vi "FPGA DAQ.vi"() -> ()   [LabVIEW 2020]
uses:
  <vilib>/Platform/TimedLoop/XDataNode/wakeup.ctl
  <vilib>/Platform/TimedLoop/XDataNode/XDNodeRunTimeDep.lvlib
  <vilib>/Platform/TimedLoop/XDataNode/nitl_modes.ctl
  <vilib>/Platform/TimedLoop/XDataNode/timing_clust.ctl
  <vilib>/Platform/TimedLoop/XDataNode/XDataNode.xnode
  <vilib>/eio/EIONode/EIONode.xnode
  <vilib>/rvi/DataTransferAndStorage/Container/XNode/niFpgaContainer.xnode
  FPGA Typedefs/Image State.ctl
  FPGA Typedefs/scan_typr.ctl
  <vilib>/rvi/interface/RandomDataEmulation/nirviRandomDataFpgaReadWriteTemplate.vi
  FPGA Typedefs/SPI Master State.ctl
  FPGA Typedefs/first_ref_frame.ctl
  <vilib>/rvi/FXPMathLib/FxpAdd/XNode/nifxpmath_Add.xnode
  <vilib>/rvi/FXPMathLib/sim/FxpSim.dll
  <vilib>/rvi/FXPMathLib/FxpMul/XNode/nifxpmath_Multiplier.xnode
  <vilib>/rvi/FXPMathLib/FxpDiv/subVIs/nifxpmath_Div_SimConfig.ctl
  <vilib>/rvi/FXPMathLib/FxpDiv/simVIs/DllFxpDivTemp_sub.vi
  <vilib>/rvi/FXPMathLib/FxpDiv/XNode/nifxpmath_Div.xnode
  <vilib>/rvi/FXPMathLib/FxpSub/XNode/nifxpmath_Sub.xnode
  <vilib>/rvi/FIFO/Fifo_Resource/niFpgaFifoEmulationRefIn.vi
  <vilib>/rvi/FIFO/Fifo_Resource/nirvififoEmulationWrite.vi
  <vilib>/rvi/FIFO/Fifo_Resource/nirvififoEmulationGetNumberOfElementsToRead.vi
  <vilib>/rvi/eio/common/nirviEmuTemplateMethod_errors.vi
  FPGA Globals/FPGA golbals.vi
  FPGA Typedefs/Stimulus trigger delays cluster.ctl
  Typedefs/Imaging Protocols enum.ctl
  FPGA Typedefs/PXI Trigger Enable cluster.ctl
  FPGA Typedefs/General trig pulse width.ctl
  Typedefs/Trigger 1 selector enum.ctl
panel:
  in  "Trigger 1 selector":T1
  out "x_offset":fxp<+/-,16,8>
  out "MC State":T2
  out "Data Out":u32
  out "_SS":bool
  in  "live_scan (triggers module)":bool
  in  "ABORT Trig loop":bool
  in  "General trig. pulse width":T3={"Trigger 1 function"=enum."Line trigger", "Pulse width (ticks)-Line Trig."=80000, "Pulse width (ticks)-Frame/Cycle Trig."=80, "Pulse width (ticks)-Trial trig."=80, "Pulse width (ticks)-Start of Exp. trig."=80000}
  in  "Experiment start":bool
  in  "var_x":fxp<+,16,4>=1.0
  in  "var_y":fxp<+,16,4>=1.0
  in  "accn_noise":fxp<+,16,16>=3200.0
  in  "use Kalman":bool
  in  "PXI Trigger Enable":T4
  in  "Imaging Protocol":T5=enum."Live Imaging"
  in  "Stimulus Trigger Setup":T6={"Trigger period in live protocols (80MHz Cycles)"=800000000, "Pulse width in live protocols (80MHz Cycles)"=40000000, "Enable stimulus in live protocols"=FALSE, "Trigger delay in funct. protocols (80MHz Cycles)"=0, "Pulse width in funct. protocols (80MHz Cycles)"=400000, "Enable stimulus in funct. protocols"=FALSE}
  in  "New line trigger enabled":bool
  in  "Ref count reset enabled":bool
  out "x_diff_PID_out":fxp<+/-,16,8>
  out "Read Value":u32
  in  "select_ref_red":bool
  out "ydiffpidvalid":bool
  out "xpiddiffvalid":bool
  out "y_diff_PID_out":fxp<+/-,16,8>
  out "y_new_ready":bool
  out "x_new_ready":bool
  in  "scan_int":fxp<+,16,2>=0.00201416015625
  in  "Integral_scale":fxp<+/-,16,12>
  in  "diff_thresh":fxp<+/-,16,8>
  in  "proportioanl_scale":fxp<+,16,2>=1.0
  in  "live_scan":bool
  in  "start":bool
  out "x_diff":fxp<+/-,16,8>
  out "y_diff":fxp<+/-,16,8>
  out "x_centroid_ref":fxp<+,32,16>
  in  "Average":u16=1
  in  "threshold":u16
  out "y_offset_u16":u16
  out "TX ready":bool
  out "y^x offset":u32
  in  "use host offset":bool
  in  "set_reference":bool
  out "x_centroid_new":fxp<+,32,16>
  out "y_centroid_new":fxp<+,32,16>
  out "y_centroid_ref":fxp<+,32,16>
  out "y_offset":fxp<+/-,16,8>
  out "x_offset_u16":u16
  in  "x_offset_host":fxp<+/-,16,8>
  in  "y_offset_host":fxp<+/-,16,8>
  in  "scale":fxp<+,16,2>=1.0
  in  "MISO":bool
  in  "RESET":bool
  in  "CPHA":bool
  in  "CPOL":bool
  in  "HCP-1":u8
  in  "add_cycle":bool
  in  "Num_pixels_slip_cycle":u32
  in  "Repeat (Number of Cycles)":u32
  in  "Mode":T7
  in  "AOD fill":u16
  in  "Ref Scan Cycles":i32=1
  in  "Start Up Delay":i32
  in  "samps-per-pix (P)":u16=1
  in  "Number-pixels-pointing (Np)":i32
  in  "Ref y-pixels-per-line (Npyr)":i16
  in  "Ref x-pixels-per-line (Npxr)":i16
  in  "Ref samps-per-pix (Pr)":u16
  in  "y-pixels-per-line (Npy)":i16
  in  "x-pixels-per-line (Npx)":i16
  in  "samples wait after trigger":u16
  # "STATE MACHINE"
  # "TRIGGERS"
  # "HANDSHAKE"
  # "MOVEMENT CORRECTION"
  # "(Trigger 5)"
  # "Many of these indicators are used in the  PC code's MC logic (in the \"Save MC Test Data.vi\"). Their values are saved to file. Eliminate if unnecessary."
  # "(80=1us)"
  # "(80=1us)"
  # "(80000=1ms)"
  # "(80000=1ms)"
  # "Limited to 53.5 sec (if U32)"
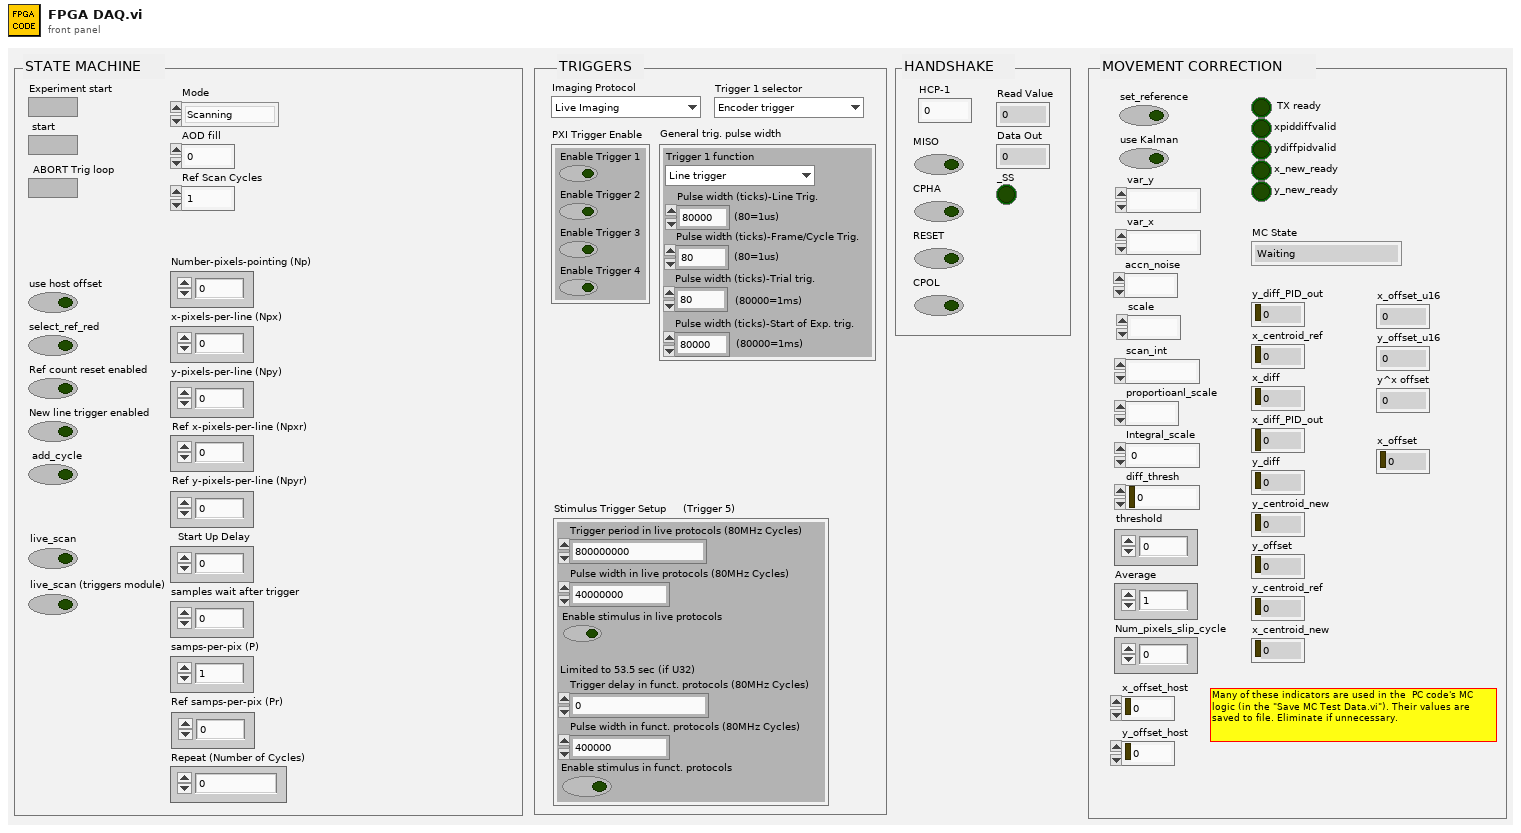
[diagram p1: front panel]
types:
  T1 = typedef "Trigger 1 selector enum.ctl" = enum16{"Encoder trigger", "Line trigger", "Control system's ref frame acknowledgement"}
  T2 = typedef "first_ref_frame.ctl" = enum16{"Waiting", "First frame", "Wrote Ref"}
  T3 = typedef "General trig pulse width.ctl" = cluster{"Trigger 1 function":T1, "Pulse width (ticks)-Line Trig.":u32, "Pulse width (ticks)-Frame/Cycle Trig.":u32, "Pulse width (ticks)-Trial trig.":u32, "Pulse width (ticks)-Start of Exp. trig.":u32}
  T4 = typedef "PXI Trigger Enable cluster.ctl" = cluster{"Enable Trigger 1":bool, "Enable Trigger 2":bool, "Enable Trigger 3":bool, "Enable Trigger 4":bool}
  T5 = typedef "Imaging Protocols enum.ctl" = enum16{"AOL Z-Stack", "Motor Z Stack", "Functional Acquisition", "Single Plane Acquisition", "Volume Acquisition", "Live Imaging", "Live Plane Imaging", "Live Volume Imaging"}
  T6 = typedef "Stimulus trigger delays cluster.ctl" = cluster{"Trigger period in live protocols (80MHz Cycles)":u32, "Pulse width in live protocols (80MHz Cycles)":u32, "Enable stimulus in live protocols":bool, "Trigger delay in funct. protocols (80MHz Cycles)":u32, "Pulse width in funct. protocols (80MHz Cycles)":u32, "Enable stimulus in funct. protocols":bool}
  T7 = typedef "scan_typr.ctl" = enum16{"Scanning", "Pointing", "Pointing & MC", "Scanning & MC"}
  T8 = typedef "Image State.ctl" = enum16{"Start Up", "Wait for Trigger", "Wait N after Trigger", "DAQ Pointing", "DAQ Scan", "Reference Scan", "Pointing AOL Fill", "Scan AOL FILL", "Reference AOL Fill"}
  T9 = typedef "XDNodeRunTimeDep.lvlib/timing_clust.ctl" = cluster{"Expected End [f-1]":u64, "Actual End [f-1]":u64, "Finished Late? [f-1]":bool, "Expected End [i-1]":u64, "Actual End [i-1]":u64, "Finished Late? [i-1]":bool, "Expected Start [i]":u64, "Actual Start [i]":u64, "Expected Start [f]":u64, "Actual Start [f]":u64, "Source Name":string, "Structure Name":string, "Period":i64, "Deadline":i64, "Offset":i64, "Start":i64, "Priority":i32, "Timeout":i32, "Mode":T10, "Wakeup Reason":T11, "Error":errorcluster, "Source Type":string, "Secondary Source Type":string, "Global End Time":u64, "Global Start Time":u64, "Frame Duration":u64, "Iteration Duration":u64, "Assigned CPU":i32, "I/O Scan Engine Mode":u32}
  T10 = typedef "XDNodeRunTimeDep.lvlib/nitl_modes.ctl" = enum32{"No Change", "Process missed periods, maintain original phase", "Discard missed periods, maintain original phase", "Process missed periods, ignore original phase", "Discard missed periods, ignore original phase"}
  T11 = typedef "XDNodeRunTimeDep.lvlib/wakeup.ctl" = enum32{"Normal", "Aborted", "Asynchronous wakeup", "Timing source error", "Timed loop error", "Timeout"}
  T12 = typedef "SPI Master State.ctl" = enum8{"RESET", "Wait for TX", "Assert MOSI", "Toggle SCLK", "Latch MISO and Toggle SCLK", "Assert MOSI and Toggle SCLK"}
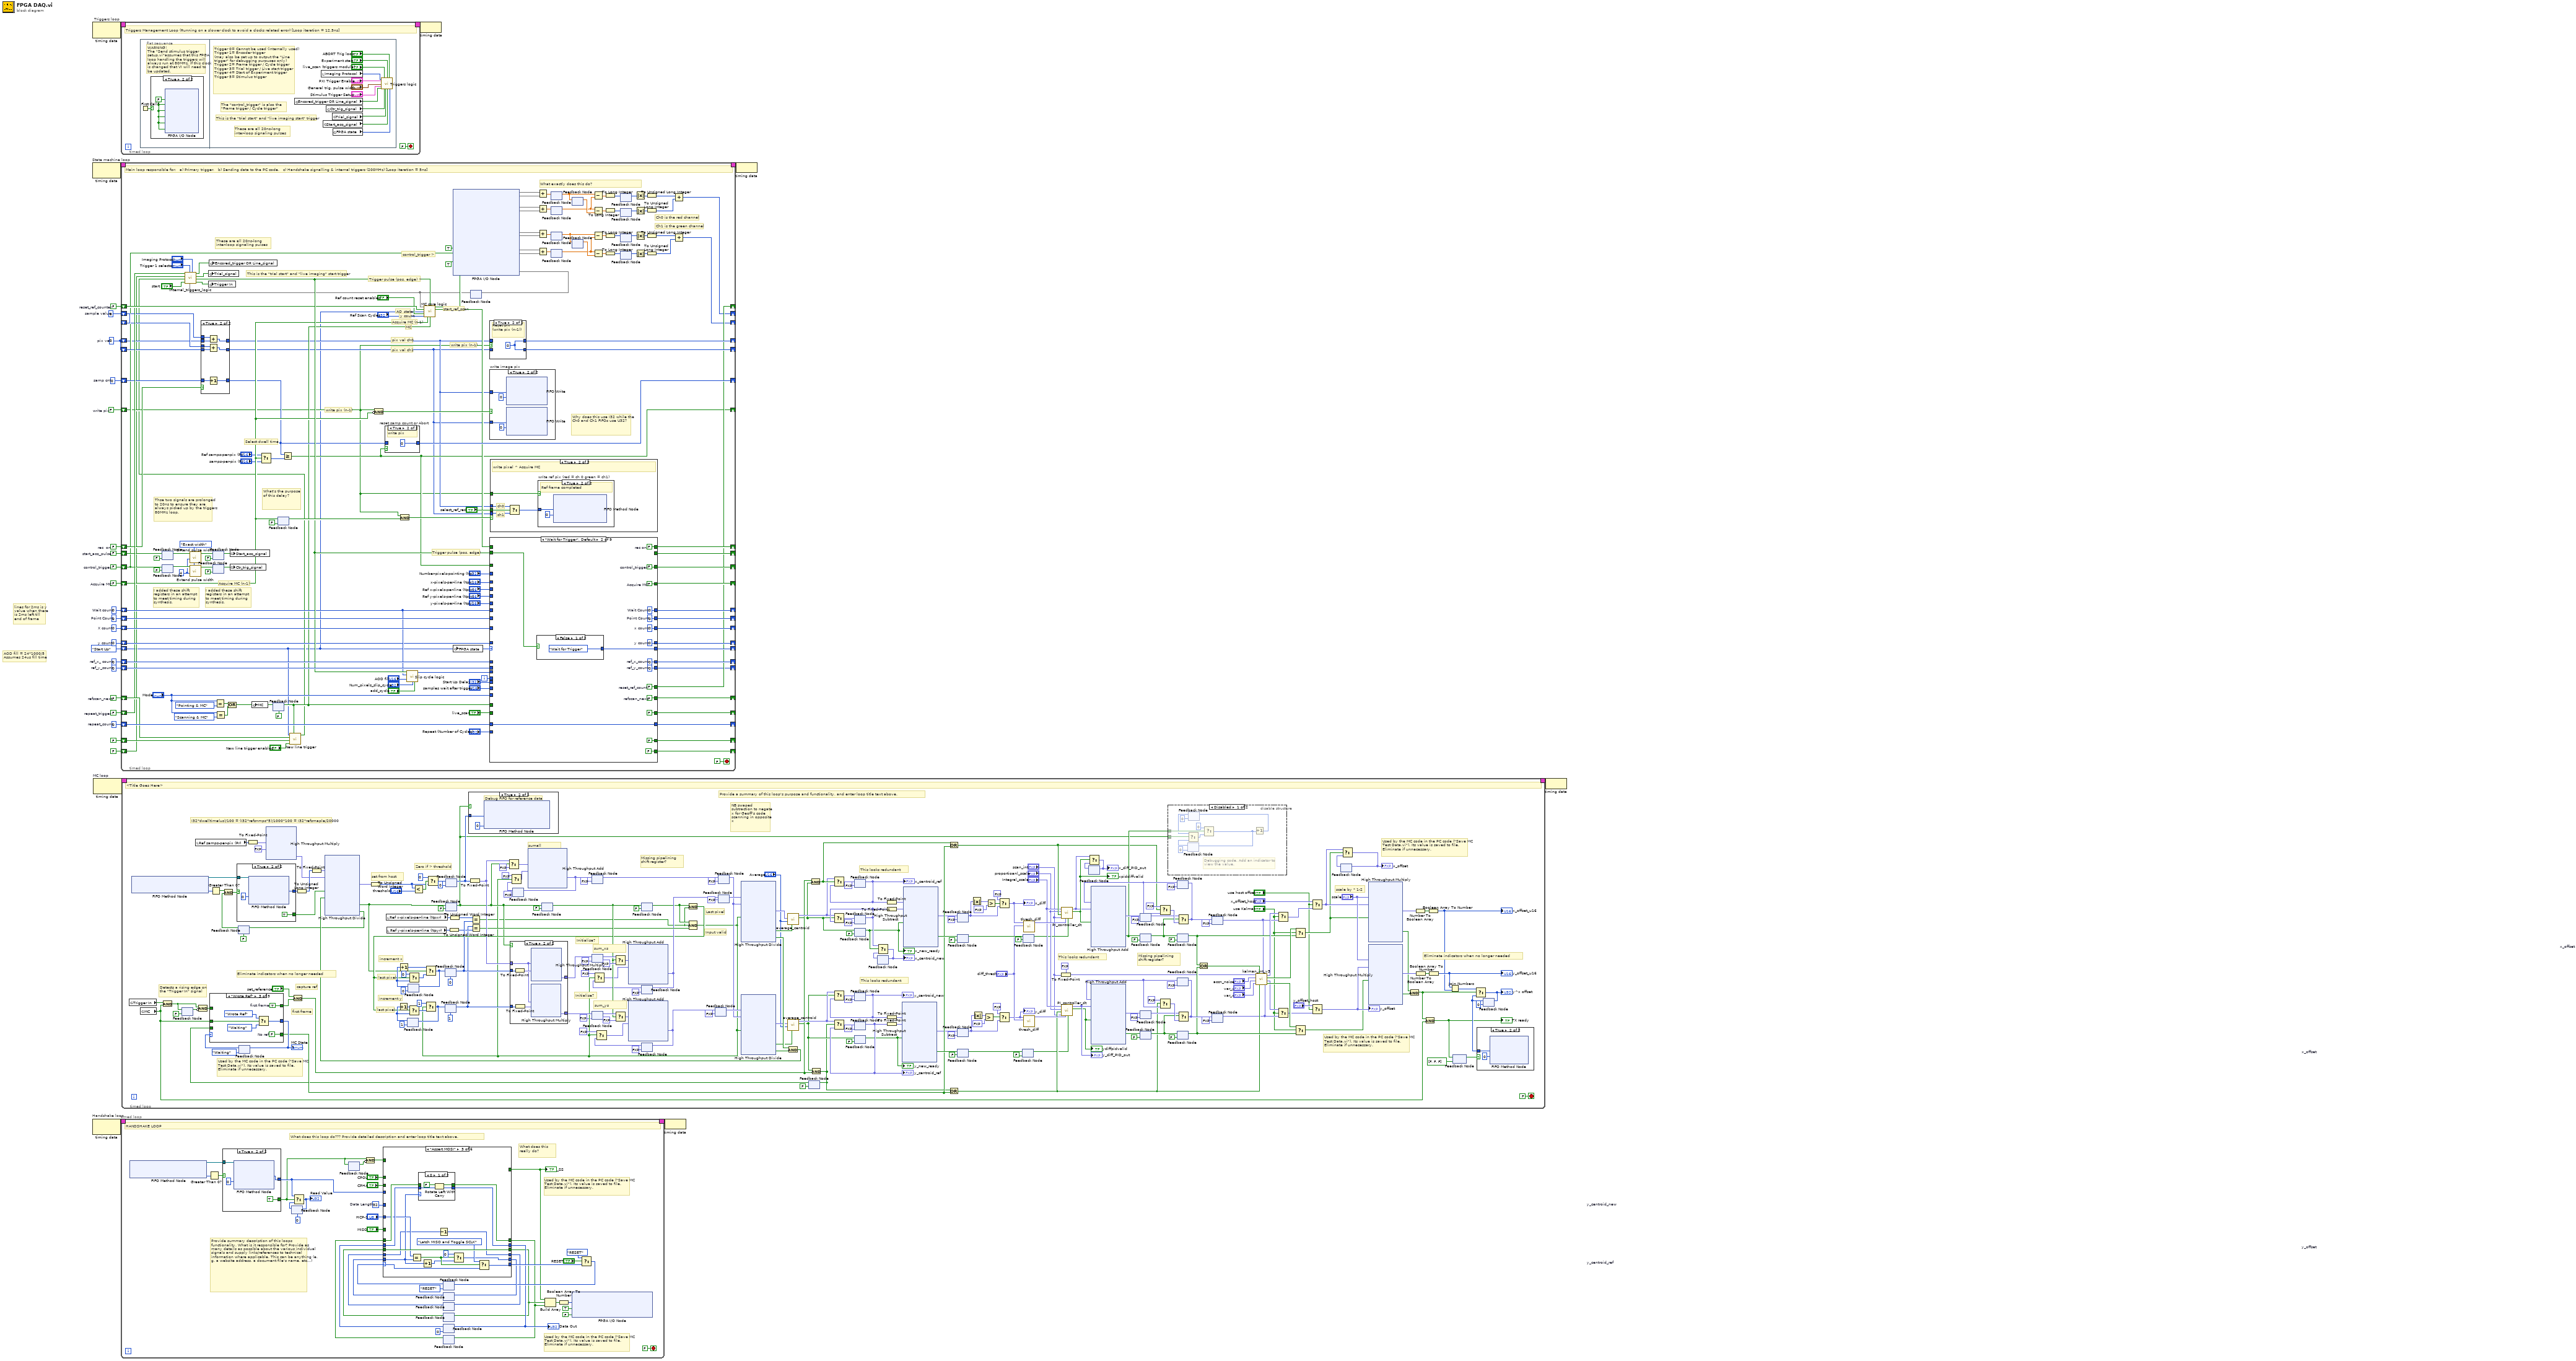
[diagram p0: block diagram]
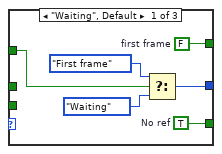
[diagram p6: hidden frame]
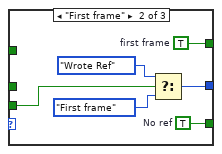
[diagram p7: hidden frame]
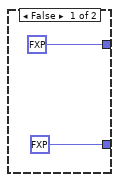
[diagram p8: hidden frame]
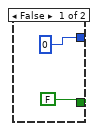
[diagram p9: hidden frame]
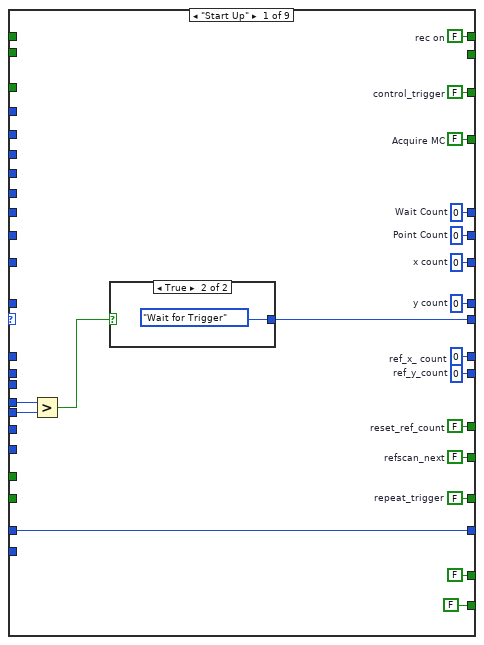
[diagram p11: hidden frame]
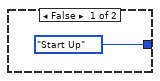
[diagram p12: hidden frame]
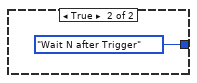
[diagram p13: hidden frame]
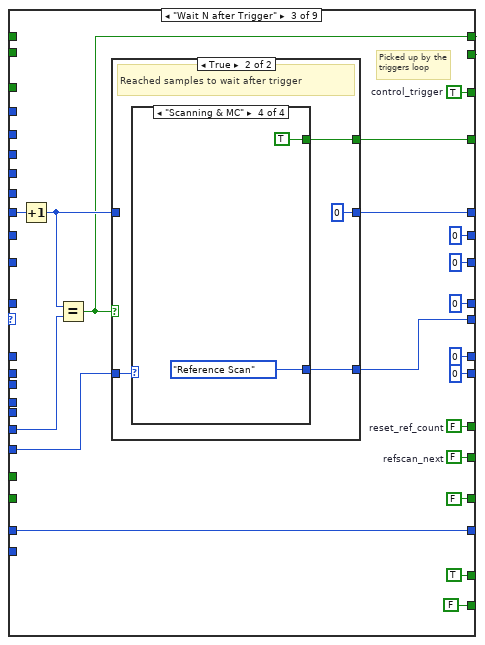
[diagram p14: hidden frame]
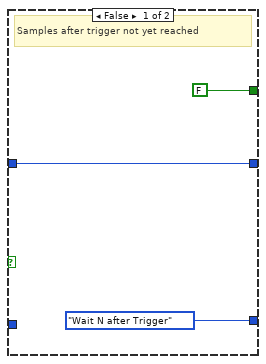
[diagram p15: hidden frame]
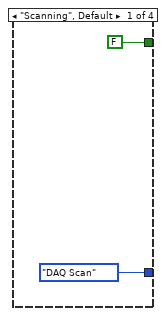
[diagram p16: hidden frame]
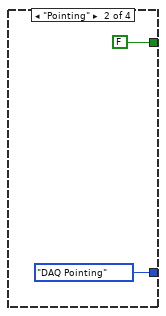
[diagram p17: hidden frame]
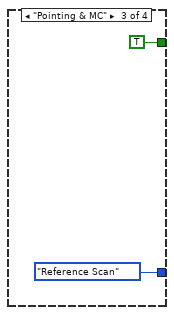
[diagram p18: hidden frame]
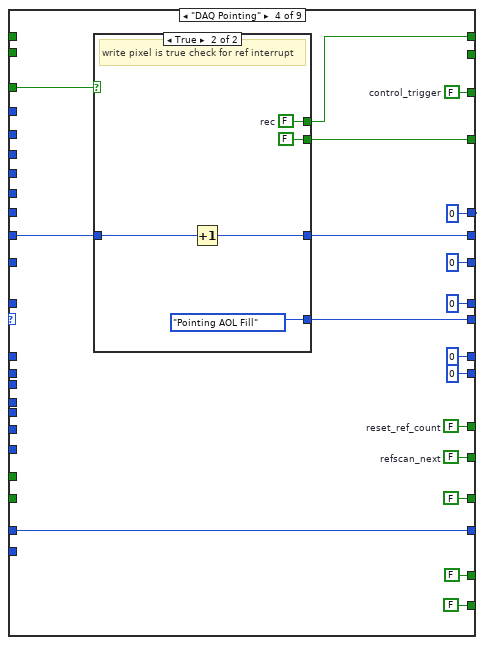
[diagram p19: hidden frame]
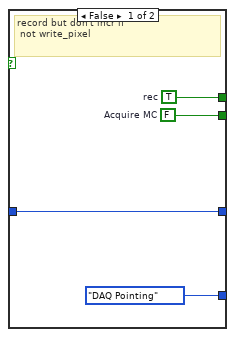
[diagram p20: hidden frame]
diagram:
  w6 = FALSE  # start_acq_pulse
  w10 = FALSE  # refscan_next
  w9 = FALSE  # reset_ref_counter
  w12 = FALSE  # repeat_trigger
  w13 = FALSE  # control_trigger
  w14 = u32 0  # repeat_count
  w16 = i16 0  # ref_y_count
  w17 = i16 0  # ref_x_ count
  w15 = u16 0  # Wait count
  w19 = FALSE  # Acquire MC
  w20 = i16 0  # y count
  w21 = i16 0  # X count
  w22 = 0  # Point Count
  w8 = FALSE  # write pix
  w7 = u32 0  # sample value
  w24 = FALSE  # rec  on
  w25 = u16 0  # samp cnt
  w23 = u32 0  # pix val
  # "lines for 2ms is y value when there is 2ms left till end of frame"
  # "AOD fill = 24*1000/5\nAssumes 24us fill time"
  n1 = node-c288() -> (w3:T9)  [unwired: 1 in]
  n2 = node-c288() -> (w27:T9)  [unwired: 1 in]
  n3 = node-c288() -> (w29:T9)  [unwired: 1 in]
  n4 = node-c288 "MC loop"() -> (w5:T9)  [unwired: 1 in]
  n5 = timed-loop "Triggers loop" {
    timing: w3 -> [_]
    timing-out: [_] -> w2
    stop <- FALSE stop-if-true
    # "Triggers Management Loop (Running on a slower clock to avoid a clocks related error) [Loop iteration = 12.5ns]"
    n6 = flat-sequence {
      frame #0 {
        # "WARNING!\nThe \"Send stimulus trigger setup.vi\"assumes that this FPGA loop handling the triggers will always run at 80MHz. If this clock is changed that VI will need to be updated."
        n7 = First Call?() -> (First Call?: T/F=w31:bool)
        n8 = case shown="True" w31 {
          frame False {
          }
          frame True {
            w32 = FALSE ("PXI_Trig0")
            n9 = xnode "FPGA I/O Node"("PXI_Trig0"=w32, "PXI_Trig1"=w32, "PXI_Trig2"=w32, "PXI_Trig3"=w32, "PXI_Trig4"=w32, "PXI_Trig5"=w32) -> ()  [unwired: 6 in, 6 out]
          }
        }
      }
      frame #1 {
        # "This is the \"trial start\" and \"live imaging start\" trigger"
        # "These are all 20ns-long inter-loop signaling pulses"
        # "The \"control_trigger\" is also the \"Frame trigger / Cycle trigger\""
        # "Trigger 0= Cannot be used (internally used)\nTrigger 1= Encoder trigger\n(may also be set up to output the \"Line trigger\" for debugging purpuses only)\nTrigger 2= Frame trigger / Cycle trigger\nTrigger 3= Trial trigger / Live start trigger\nTrigger 4= Start of Experiment trigger\nTrigger 5= Stimulus trigger"
        n10 = global read "FPGA golbals.vi" "Encored_trigger OR Line_signal"() -> (w36:bool)
        n11 = local read "Imaging Protocol"() -> (w33:T5)
        n12 = global read "FPGA golbals.vi" "Start_acq_signal"() -> (w38:bool)
        n13 = global read "FPGA golbals.vi" "Ctr_trig_signal"() -> (w37:bool)
        n14 = global read "FPGA golbals.vi" "Trial_signal"() -> (w39:bool)
        n15 = global read "FPGA golbals.vi" "FPGA state"() -> (w34:T8)
        n16 = call "Triggers logic.vi"("Imaging Protocol"=w33, "PXI Trigger Enable"="PXI Trigger Enable", "General trig. pulse width"="General trig. pulse width", "Stimulus Trigger Setup"="Stimulus Trigger Setup", "Encored_trigger OR Line_signal"=w36, "live_scan"="live_scan (triggers module)", "Ctr_trig_signal"=w37, "Trial_signal"=w39, "Experiment start"="Experiment start", "Start_acq_signal"=w38, "Abort triggers"="ABORT Trig loop", "FPGA state"=w34) -> ()  [unwired: 7 in, 1 out]
      }
    }
  }
  n17 = timed-loop "State machine loop" {
    timing: w27 -> [_]
    timing-out: [_] -> w26
    shift-right: [w191] -> _
    shift-left: w23 -> [w153]
    shift-right: [w193] -> _
    shift-left: w25 -> [w152]
    shift-right: [w100] -> _
    shift-left: w7 -> [w154]
    shift-right: [w102] -> _
    shift-left: w8 -> [w96]
    shift-right: [w130] -> _
    shift-left: w24 -> [w162]
    shift-right: [w101] -> _
    shift-left: w7 -> [w115]
    shift-right: [w192] -> _
    shift-left: w23 -> [w99]
    shift-right: [w125] -> _
    shift-left: Image_State."Start Up" ("Enum") -> [w48]
    shift-right: [w123] -> _
    shift-left: w22 -> [w188]
    shift-right: [w121] -> _
    shift-left: w21 -> [w189]
    shift-right: [w124] -> _
    shift-left: w20 -> [w164]
    shift-right: [w128] -> _
    shift-left: w19 -> [w137]
    shift-right: [w126] -> _
    shift-left: w17 -> [w186]
    shift-right: [w111] -> _
    shift-left: w16 -> [w187]
    shift-right: [w122] -> _
    shift-left: w15 -> [w166]
    shift-right: [w117] -> _
    shift-left: w14 -> [w181]
    shift-right: [w129] -> _
    shift-left: w13 -> [w108]
    shift-right: [w118] -> _
    shift-left: w12 -> [w163]
    shift-right: [w116] -> _
    shift-left: FALSE -> [w177]
    shift-right: [w120] -> _
    shift-left: w9 -> [w165]
    shift-right: [w119] -> _
    shift-left: w10 -> [w178]
    shift-right: [w127] -> _
    shift-left: w6 -> [w160]
    shift-right: [w55] -> _
    shift-left: FALSE -> [w53]
    i -> [w190]
    stop <- FALSE stop-if-true
    w161 = enum16{"Minimum width", "Exact width"}."Exact width" ("Function")
    w151 = u32 4 ("Pulse width (ticks)(80000=1ms @80MHz)")
    # "These are all 20ns-long inter-loop signaling pulses"
    # "This is the \"trial start\" and \"live imaging\" start trigger"
    # "What exactly does this do?"
    # "Ch1 is the green channel"
    # "Ch0 is the red channel"
    # "write pix (n-1)"
    # "pix val ch1"
    # "pix val ch0"
    # "control_trigger >"
    # "What's the purpose of this delay?"
    # "write pix (n-1)"
    # "Why does this use I32 while the Ch0 and Ch1 FIFOs use U32?"
    # "Select dwell time"
    # "Trigger pulse (pos. edge)"
    # "I added these shift registers in an attempt to meet timing during synthesis."
    # "I added these shift registers in an attempt to meet timing during synthesis."
    # "Thse two signals are prolonged to 20ns to ensure they are always picked up by the triggers 80MHz loop."
    # "MC"
    # "AQ_state"
    # "Trigger pulse (pos. edge) >"
    # "Acquire MC (n-1)"
    # "start_ref_scan"
    # "Acquire MC (n-1)"
    # "y count"
    # "Main loop responsible for:   a) Primary trigger,   b) Sending data to the PC code,   c) Handshake signalling & internal triggers (200MHz) [Loop iteration = 5ns]"
    n18 = feedback #1(FALSE ("Acquire MC")) -> (w159:bool)
    n19 = feedback-in #1(w160) -> ()
    n20 = feedback #2(FALSE ("Acquire MC")) -> (w158:bool)
    n21 = feedback-in #2(w108) -> ()
    n22 = call "Extend pulse width.vi"("Function"=w161, "Pulse width (ticks)(80000=1ms @80MHz)"=w151, "Input signal"=w159) -> ("Output signal"=w157:bool)  [unwired: 8 in]
    n23 = call "Extend pulse width.vi"("Function"=w161, "Pulse width (ticks)(80000=1ms @80MHz)"=w151, "Input signal"=w158) -> ("Output signal"=w156:bool)  [unwired: 8 in]
    n24 = case shown="True" w162 {
      tunnel: w153 -> [w196 w204]
      tunnel: [w196 w203] -> w97
      tunnel: w152 -> [w195 w202]
      tunnel: [w195 w201] -> w113
      tunnel: w154 -> [_ w200]
      tunnel: w99 -> [w194 w199]
      tunnel: w115 -> [_ w198]
      tunnel: [w194 w197] -> w98
      frame False {
      }
      frame True {
        n25 = Add(x=w198, y=w199) -> (x+y=w197:u32)
        n26 = Add(x=w200, y=w204) -> (x+y=w203:u32)
        n27 = Increment(x=w202) -> (x+1=w201:u16)
      }
    }
    n28 = feedback #3(FALSE ("Acquire MC")) -> (w105:bool)
    n29 = feedback-in #3(w157) -> ()
    n30 = feedback #4(FALSE ("Acquire MC")) -> (w104:bool)
    n31 = feedback-in #4(w156) -> ()
    n32 = Equal?(x="Mode", y=scan_typr."Pointing & MC" ("Mode 2")) -> (x = y?=w183:bool)
    n33 = Equal?(x="Mode", y=scan_typr."Scanning & MC" ("Mode 2")) -> (x = y?=w182:bool)
    n34 = Or(x=w183, y=w182) -> (x .or. y?=w103:bool)
    n35 = global write "FPGA golbals.vi" "Start_acq_signal"(w105) -> ()
    n36 = global write "FPGA golbals.vi" "Ctr_trig_signal"(w104) -> ()
    n37 = global write "FPGA golbals.vi" "MC"(w103) -> ()
    n38 = Select(t="Ref samps-per-pix (Pr)", s=w137, f="samps-per-pix (P)") -> (s? t:f=w114:u16)
    n39 = feedback-in #5(w103) -> ()
    n40 = feedback #5(FALSE ("Acquire MC")) -> (w112:bool)
    n41 = feedback #6(FALSE ("Acquire MC")) -> (w174:bool)
    n42 = feedback-in #6(w137) -> ()
    n43 = Greater Or Equal?(x=w113, y=w114) -> (x >= y?=w102:bool)
    n44 = call "New line trigger.vi"("MC"=w112, "New line trigger enabled"="New line trigger enabled", "aod_fill_active in"=w177, "refscan_next"=w178, "AQ STATE"=w48) -> ("aod_fill_active"=w51:bool)  [unwired: 6 in]
    n45 = Compound Arithmetic op=AND(w96, invert w137) -> (w179:bool)
    n46 = case "reset samp count or Abort" shown="True" w102 {
      tunnel: [w609 u16 0] -> w193
      tunnel: w113 -> [w609 _]
      frame False {
      }
      frame True {
        # "write pix"
      }
    }
    n47 = And(x=w96, y=w174) -> (x .and. y?=w173:bool)
    n48 = global write "FPGA golbals.vi" "FPGA state"(w48) -> ()
    n49 = feedback #7() -> (w49)  [unwired: 1 in]
    n50 = call "Internal_triggers_logic.vi"("Imaging Protocol"="Imaging Protocol", "aol_ref_scan_next"=w49, "Trigger 1 selector"="Trigger 1 selector", "Start"="start", "Line_signal"=w51, "End of trial"=w53, "Repeat trigger"=w163) -> ("Trigger In"=w106:bool, "Trigger pulse (pos. edge)"=w169:bool, "Trial start trigger signal"=w107:bool, "Encoder trigger signal"=w52:bool)  [unwired: 1 in]
    n51 = global write "FPGA golbals.vi" "Trial_signal"(w107) -> ()
    n52 = global write "FPGA golbals.vi" "Trigger In"(w106) -> ()
    n53 = global write "FPGA golbals.vi" "Encored_trigger OR Line_signal"(w52) -> ()
    n54 = call "Slip cycle logic.vi"("Trigger pulse (pos. edge)"=w169, "Wait Count"=w166, "AOD fill in"="AOD fill", "Num_pixels_slip_cycle"="Num_pixels_slip_cycle", "add_cycle"="add_cycle") -> ("AOD fill out"=w171:u16)  [unwired: 10 in]
    n55 = call "MC core logic.vi"("AOL_ref_scan_next"=w49, "Trigger pulse (pos. edge)"=w169, "Reset_ref_counter"=w165, "State"=w48, "Ref count reset enabled"="Ref count reset enabled", "Ref Scan Cycles"="Ref Scan Cycles", "Acquire MC"=w137, "MC"=w112) -> ("start_aol_ref_scan"=w109:bool, "start_ref_scan"=w131:bool)  [unwired: 6 in]
    n56 = xnode ("FPGA I/O Node")("IO Module\\Trigger WE"=TRUE ("IO Module\\Trigger WE"), "IO Module\\Trigger Output"=w108, "IO Module\\PFI 0 Wr Data"=w109, "IO Module\\PFI 0 WE"=TRUE ("IO Module\\PFI 0 WE")) -> ("IO Module\\AI 0 Data N"=w93, "IO Module\\AI 0 Data N-1"=w92, "IO Module\\AI 0 Data N-2"=w91, "IO Module\\AI 0 Data N-3"=w90, "IO Module\\AI 1 Data N"=w89, "IO Module\\AI 1 Data N-1"=w88, "IO Module\\AI 1 Data N-2"=w87, "IO Module\\AI 1 Data N-3"=w86, "IO Module\\PFI 1 Rd Data"=w110)  [unwired: 13 in, 13 out]
    n57 = feedback-in #7(w110) -> ()
    n58 = case shown="True" w96 {
      tunnel: [w612 w613] -> w191
      tunnel: w97 -> [w612 _]
      tunnel: w98 -> [w611 _]
      tunnel: [w611 w613] -> w192
      frame False {
      }
      frame True {
        w613 = u32 0
        # "Reset pix\n(write pix (n-1))"
      }
    }
    n59 = case "write image pix" shown="True" w179 {
      tunnel: w98 -> [_ w608]
      tunnel: w97 -> [_ w606]
      frame False {
      }
      frame True {
        n60 = xnode ("FIFO Write")("Element"=w608, "Timeout"=0) -> ()  [unwired: 1 in, 2 out]
        n61 = xnode ("FIFO Write")("Element"=w606, "Timeout"=0) -> ()  [unwired: 1 in, 2 out]
      }
    }
    n62 = case shown="\"Wait for Trigger\", Default" w48 {
      tunnel: w190 -> [w223 _ _ _ _ _ _ _ _]
      tunnel: "Start Up Delay" -> [w222 _ _ _ _ _ _ _ _]
      tunnel: [w220 w237 w262 w288 w323 w376 w439 w508 w569] -> w125
      tunnel: [w219 w241 w246 w289 w318 w378 w438 w507 w565] -> w130
      tunnel: [w218 w240 0 ("x count") w291 0 ("x count") w361 w432 0 ("x count") w567] -> w123
      tunnel: w188 -> [_ _ _ w292 _ w362 w423 _ w567]
      tunnel: [w217 w239 i16 0 i16 0 ("x count") w321 w359 i16 0 ("x count") w492 w574] -> w121
      tunnel: w189 -> [_ _ _ _ w319 w360 _ w493 w574]
      tunnel: [w216 w238 i16 0 i16 0 ("y count") w322 w357 i16 0 ("y count") w501 w570] -> w124
      tunnel: w164 -> [_ _ _ _ w320 w358 _ w490 w570]
      tunnel: [w215 w242 w247 w290 w317 w356 w437 w506 w564] -> w128
      tunnel: "samples wait after trigger" -> [_ _ w264 _ _ _ _ _ _]
      tunnel: "Mode" -> [_ _ w259 _ _ _ _ _ w563]
      tunnel: w169 -> [_ w236 _ _ _ _ _ _ _]
      tunnel: "Number-pixels-pointing (Np)" -> [_ _ _ _ _ _ w424 _ _]
      tunnel: w112 -> [_ _ _ _ _ _ w434 w503 _]
      tunnel: [w214 w235 w258 u16 0 ("Wait Count") u16 0 ("Wait count") u16 0 ("Wait count") w442 w511 w573] -> w122
      tunnel: w171 -> [_ _ _ _ _ _ w443 w510 w572]
      tunnel: w131 -> [_ _ _ _ _ _ w433 w502 _]
      tunnel: "x-pixels-per-line (Npx)" -> [_ _ _ _ w310 _ _ _ _]
      tunnel: "y-pixels-per-line (Npy)" -> [_ _ _ _ _ _ _ w491 _]
      tunnel: "Ref x-pixels-per-line (Npxr)" -> [_ _ _ _ _ w364 _ _ _]
      tunnel: "Ref y-pixels-per-line (Npyr)" -> [_ _ _ _ _ _ _ _ w557]
      tunnel: [w213 w234 i16 0 ("Wait count") i16 0 ("Wait count") i16 0 ("Wait count") w374 i16 0 ("ref_x_count") i16 0 ("ref_x_count") w568] -> w126
      tunnel: [w212 w233 i16 0 ("ref_y_count") i16 0 ("ref_y_count") i16 0 ("ref_y_count") w373 i16 0 ("ref_y_count") i16 0 ("ref_y_count") w556] -> w111
      tunnel: w187 -> [_ _ _ _ _ w372 _ _ w556]
      tunnel: w186 -> [_ _ _ _ _ w371 _ _ w568]
      tunnel: w166 -> [_ _ w254 _ _ _ w417 w488 w554]
      tunnel: "Repeat (Number of Cycles)" -> [_ _ _ _ _ _ w421 w486 _]
      tunnel: w181 -> [w211 w232 w253 w287 w316 w370 w418 w484 w566]
      tunnel: [w211 w232 w253 w287 w316 w370 w431 w500 w566] -> w117
      tunnel: [w210 w231 w252 w286 w315 w369 w430 w499 w562] -> w129
      tunnel: [w209 FALSE FALSE FALSE FALSE FALSE w429 w498 FALSE] -> w118
      tunnel: "live_scan" -> [_ _ _ _ _ _ w428 w497 _]
      tunnel: [FALSE FALSE TRUE FALSE FALSE FALSE TRUE TRUE TRUE] -> w116
      tunnel: [w207 w228 w249 w283 w312 w366 w426 w495 w559] -> w120
      tunnel: [w206 w227 w248 w282 w311 w365 w425 w494 w558] -> w119
      tunnel: [_ _ w246 _ _ _ _ _ _] -> w127
      tunnel: w102 -> [_ _ _ w281 w308 w355 _ _ _]
      tunnel: [FALSE FALSE FALSE FALSE FALSE FALSE w415 w482 FALSE] -> w55
      frame "Start Up" {
        w206 = FALSE  # refscan_next
        w207 = FALSE  # reset_ref_count
        w209 = FALSE  # repeat_trigger
        w210 = FALSE  # control_trigger
        w212 = i16 0  # ref_y_count
        w213 = i16 0  # ref_x_ count
        w214 = u16 0  # Wait Count
        w215 = FALSE  # Acquire MC
        w216 = i16 0  # y count
        w217 = i16 0  # x count
        w219 = FALSE  # rec on
        w218 = 0  # Point Count
        n63 = Greater?(x=w223, y=w222) -> (0:w221:bool)
        n64 = case shown="True" w221 {
          tunnel: [Image_State."Start Up" Image_State."Wait for Trigger"] -> w220
          frame False {
          }
          frame True {
          }
        }
      }
      frame "Wait for Trigger", Default {
        w227 = FALSE  # refscan_next
        w228 = FALSE  # reset_ref_count
        w231 = FALSE  # control_trigger
        w233 = i16 0  # ref_y_count
        w234 = i16 0  # ref_x_count
        w235 = u16 0  # Wait Count
        w242 = FALSE  # Acquire MC
        w238 = i16 0  # y count
        w239 = i16 0  # x count
        w241 = FALSE  # rec on
        w240 = 0  # Point Count
        n65 = case shown="False" w236 {
          tunnel: [Image_State."Wait for Trigger" Image_State."Wait N after Trigger"] -> w237
          frame False {
          }
          frame True {
          }
        }
      }
      frame "Wait N after Trigger" {
        w248 = FALSE  # refscan_next
        w249 = FALSE  # reset_ref_count
        w252 = TRUE  # control_trigger
        # "Picked up by the triggers loop"
        # "time includes AOD fill time"
        n66 = Increment(x=w254) -> (x+1=w263:u16)
        n67 = Equal?(x=w263, y=w264) -> (x = y?=w246:bool)
        n68 = case shown="True" w246 {
          tunnel: w263 -> [w267 _]
          tunnel: [w267 u16 0] -> w258
          tunnel: [Image_State."Wait N after Trigger" w269] -> w262
          tunnel: [FALSE w270] -> w247
          tunnel: w259 -> [_ w268]
          frame False {
            # "Samples after trigger not yet reached"
          }
          frame True {
            # "Reached samples to wait after trigger"
            n69 = case shown="\"Scanning & MC\"" w268 {
              tunnel: [FALSE FALSE TRUE TRUE] -> w270
              tunnel: [Image_State."DAQ Scan" Image_State."DAQ Pointing" Image_State."Reference Scan" Image_State."Reference Scan"] -> w269
              frame "Scanning", Default {
              }
              frame "Pointing" {
              }
              frame "Pointing & MC" {
              }
              frame "Scanning & MC" {
              }
            }
          }
        }
      }
      frame "DAQ Pointing" {
        w282 = FALSE  # refscan_next
        w283 = FALSE  # reset_ref_count
        w286 = FALSE  # control_trigger
        n70 = case shown="True" w281 {
          tunnel: [Image_State."DAQ Pointing" ("Enum") Image_State."Pointing AOL Fill" ("Enum")] -> w288
          tunnel: [w300 w306] -> w289
          tunnel: [w298 w305] -> w291
          tunnel: [w299 FALSE] -> w290
          tunnel: w292 -> [w298 w304]
          frame False {
            w299 = FALSE  # Acquire MC
            w300 = TRUE  # rec
            # "record but don't incr if \n not write_pixel"
          }
          frame True {
            w306 = FALSE  # rec
            # "write pixel is true check for ref interrupt"
            n71 = Increment(x=w304) -> (x+1=w305:i32)
          }
        }
      }
      frame "DAQ Scan" {
        w311 = FALSE  # refscan_next
        w312 = FALSE  # reset_ref_count
        w315 = FALSE  # control_trigger
        n72 = Decrement(x=w310) -> (x-1=w309:i16)
        n73 = Equal?(x=w309, y=w319) -> (x = y?=w324:bool)
        n74 = case shown="True" w308 {
          tunnel: [w333 w336] -> w318
          tunnel: [FALSE w335] -> w317
          tunnel: w319 -> [w331 w341]
          tunnel: [w331 w340] -> w321
          tunnel: w320 -> [w330 w339]
          tunnel: [w330 w338] -> w322
          tunnel: [Image_State."DAQ Scan" ("Enum") w337] -> w323
          tunnel: w324 -> [_ w334]
          frame False {
            w333 = TRUE  # rec
            # "accumulate samples for pixel"
          }
          frame True {
            # "write pixel check for  end of line"
            n75 = case shown="True" w334 {
              tunnel: w341 -> [w347 _]
              tunnel: [w346 w353] -> w340
              tunnel: w339 -> [w345 w352]
              tunnel: [w345 w351] -> w338
              tunnel: [Image_State."DAQ Scan" ("Enum") Image_State."Scan AOL FILL" ("Enum")] -> w337
              tunnel: [w343 w350] -> w336
              tunnel: [w342 w349] -> w335
              frame False {
                w342 = FALSE  # Acq MC
                w343 = TRUE  # rec
                # "not end of line"
                n76 = Increment(x=w347) -> (x+1=w346:i16)
              }
              frame True {
                w349 = FALSE  # Acquire MC
                w350 = FALSE  # rec
                w353 = i16 0  # x count
                # "End of line"
                n77 = Increment(x=w352) -> (x+1=w351:i16)
              }
            }
          }
        }
      }
      frame "Reference Scan" {
        w356 = TRUE  # Acq MC
        w365 = FALSE  # refscan_next
        w366 = FALSE  # reset_ref_count
        w369 = FALSE  # control_trigger
        n78 = Decrement(x=w364) -> (x-1=w363:i16)
        n79 = Equal?(x=w363, y=w371) -> (x = y?=w375:bool)
        n80 = case shown="True" w355 {
          tunnel: [w385 w396] -> w378
          tunnel: [Image_State."Reference Scan" ("Enum") w397] -> w376
          tunnel: w375 -> [_ w398]
          tunnel: w371 -> [w383 w395]
          tunnel: [w383 w394] -> w374
          tunnel: w372 -> [w382 w393]
          tunnel: [w382 w392] -> w373
          tunnel: w362 -> [w381 w391]
          tunnel: [w381 w390] -> w361
          tunnel: w360 -> [w380 w389]
          tunnel: [w380 w388] -> w359
          tunnel: w358 -> [w379 w387]
          tunnel: [w379 w386] -> w357
          frame False {
            w385 = TRUE  # rec
            # "accumulate samples for pixel"
          }
          frame True {
            # "write pixel check for  end of line"
            n81 = case shown="False" w398 {
              tunnel: [w406 i16 0] -> w394
              tunnel: [Image_State."Reference Scan" ("Enum") Image_State."Reference AOL Fill" ("Enum")] -> w397
              tunnel: [w405 w410] -> w396
              tunnel: w395 -> [w404 _]
              tunnel: w393 -> [w403 w413]
              tunnel: [w403 w412] -> w392
              tunnel: [w401 w409] -> w390
              tunnel: w391 -> [w401 w409]
              tunnel: [w400 w408] -> w388
              tunnel: w389 -> [w400 w408]
              tunnel: [w399 w407] -> w386
              tunnel: w387 -> [w399 w407]
              frame False {
                w405 = TRUE  # rec
                # "not end of line"
                n82 = Increment(x=w404) -> (x+1=w406:i16)
              }
              frame True {
                w410 = FALSE  # rec
                # "end of line - AOL Fill"
                n83 = Increment(x=w413) -> (x+1=w412:i16)
              }
            }
          }
        }
      }
      frame "Pointing AOL Fill" {
        w430 = FALSE  # control_trigger
        n84 = And(x=w433, y=w434) -> (x .and. y?=w425:bool)
        n85 = Equal?(x=w424, y=w423) -> (x = y?=w422:bool)
        n86 = Equal?(x=w417, y=w443) -> (x = y?=w438:bool)
        n87 = Increment(x=w418) -> (x+1=w419:u32)
        n88 = Greater Or Equal?(x=w418, y=w421) -> (x >= y?=w420:bool)
        n89 = Increment(x=w417) -> (x+1=w416:u16)
        n90 = case shown="True" w438 {
          tunnel: [w464 w475] -> w442
          tunnel: [w462 w472] -> w439
          tunnel: [FALSE ("Acquire MC") w474] -> w437
          tunnel: w425 -> [_ w473]
          tunnel: w416 -> [w445 _]
          tunnel: w423 -> [w449 w471]
          tunnel: [w460 w471] -> w432
          tunnel: w421 -> [_ _]
          tunnel: w418 -> [w457 w470]
          tunnel: [w458 w470] -> w431
          tunnel: [w450 FALSE] -> w429
          tunnel: w428 -> [w455 _]
          tunnel: [w452 w468] -> w426
          tunnel: w422 -> [w448 _]
          tunnel: w420 -> [w447 _]
          tunnel: w419 -> [w446 _]
          tunnel: [w444 FALSE] -> w415
          frame False {
            w452 = FALSE  # reset_ref_count
            # "counting AOD fill time and check for last"
            n91 = Select(t=w446, s=w448, f=w457) -> (s? t:f=w456:u32)
            n92 = Compound Arithmetic op=AND(w448, w455) -> (w454:bool)
            n93 = Compound Arithmetic op=AND(w448, invert w447) -> (w453:bool)
            n94 = Compound Arithmetic op=AND(w448, w447) -> (w444:bool)
            n95 = Or(x=w454, y=w453) -> (x .or. y?=w450:bool)
            n96 = Select(t=u32 0, s=w444, f=w456) -> (s? t:f=w458:u32)
            n97 = Select(t=Image_State."Wait for Trigger" ("Enum"), s=w448, f=Image_State."Pointing AOL Fill" ("Enum")) -> (s? t:f=w462:T8)
            n98 = Select(t=u16 0, s=w448, f=w445) -> (s? t:f=w464:u16)
            n99 = Select(t=0, s=w448, f=w449) -> (s? t:f=w460:i32)
          }
          frame True {
            w475 = u16 0  # Wait count
            # "AOD fill time reached check to see if ref scan interrupt"
            n100 = case shown="True" w473 {
              tunnel: [Image_State."DAQ Pointing" ("Enum") Image_State."Reference Scan" ("Enum")] -> w472
              tunnel: [FALSE ("Acquire MC") TRUE ("Acquire MC")] -> w474
              tunnel: [w476 w479] -> w468
              frame False {
                w476 = FALSE  # reset_ref_count
              }
              frame True {
                w479 = TRUE  # reset_ref_count
                # "scan interrupt\nset AcquireMC"
              }
            }
          }
        }
      }
      frame "Scan AOL FILL" {
        w499 = FALSE  # control_trigger
        n101 = And(x=w502, y=w503) -> (x .and. y?=w494:bool)
        n102 = Increment(x=w488) -> (x+1=w487:u16)
        n103 = Equal?(x=w491, y=w490) -> (x = y?=w489:bool)
        n104 = Equal?(x=w488, y=w510) -> (x = y?=w507:bool)
        n105 = Increment(x=w484) -> (x+1=w483:u32)
        n106 = Greater Or Equal?(x=w484, y=w486) -> (x >= y?=w485:bool)
        n107 = case shown="True" w507 {
          tunnel: [w531 w545] -> w511
          tunnel: [w534 w544] -> w508
          tunnel: w494 -> [_ w543]
          tunnel: [w535 w542] -> w506
          tunnel: w487 -> [w516 _]
          tunnel: w490 -> [w518 w541]
          tunnel: [w530 w541] -> w501
          tunnel: w484 -> [w520 w540]
          tunnel: w486 -> [_ _]
          tunnel: [w526 w540] -> w500
          tunnel: [w519 w539] -> w498
          tunnel: w497 -> [w524 _]
          tunnel: [w521 w538] -> w495
          tunnel: w493 -> [w517 w537]
          tunnel: [w517 w537] -> w492
          tunnel: w489 -> [w515 _]
          tunnel: w485 -> [w514 _]
          tunnel: w483 -> [w513 _]
          tunnel: [w512 FALSE] -> w482
          frame False {
            w521 = FALSE  # reset_ref_count
            w535 = FALSE  # Acquire MC
            # "counting AOD fill time and check finished last line"
            n108 = And(x=w515, y=w514) -> (x .and. y?=w512:bool)
            n109 = And(x=w515, y=w524) -> (x .and. y?=w523:bool)
            n110 = Compound Arithmetic op=AND(w515, invert w514) -> (w522:bool)
            n111 = Or(x=w523, y=w522) -> (x .or. y?=w519:bool)
            n112 = Select(t=Image_State."Wait for Trigger" ("Enum"), s=w515, f=Image_State."Scan AOL FILL" ("Enum")) -> (s? t:f=w534:T8)
            n113 = Select(t=w513, s=w515, f=w520) -> (s? t:f=w527:u32)
            n114 = Select(t=u16 0, s=w515, f=w516) -> (s? t:f=w531:u16)
            n115 = Select(t=i16 0, s=w515, f=w518) -> (s? t:f=w530:i16)
            n116 = Select(t=u32 0, s=w512, f=w527) -> (s? t:f=w526:u32)
          }
          frame True {
            w539 = FALSE  # repeat_trigger
            w545 = u16 0  # Wait count
            # "AOD fill time reached check to see if ref scan interrupt"
            n117 = case shown="True" w543 {
              tunnel: [Image_State."DAQ Scan" ("Enum") Image_State."Reference Scan" ("Enum")] -> w544
              tunnel: [w548 w550] -> w542
              tunnel: [w546 w549] -> w538
              frame False {
                w546 = FALSE  # reset_ref_count
                w548 = FALSE  # Acquire MC
                # "resume scan"
              }
              frame True {
                w549 = TRUE  # reset_ref_count
                w550 = TRUE  # Acquire MC
                # "scan interrupt\nset AcquireMC"
              }
            }
          }
        }
      }
      frame "Reference AOL Fill" {
        w558 = FALSE  # refscan_next
        w559 = FALSE  # reset_ref_count
        w562 = FALSE  # control_trigger
        n118 = Equal?(x=w554, y=w572) -> (x = y?=w571:bool)
        n119 = Equal?(x=w557, y=w556) -> (x = y?=w555:bool)
        n120 = Increment(x=w554) -> (x+1=w553:u16)
        n121 = case shown="True" w571 {
          tunnel: [w575 w584] -> w573
          tunnel: [Image_State."Reference AOL Fill" ("Enum") w583] -> w569
          tunnel: w553 -> [w575 _]
          tunnel: [w577 w582] -> w565
          tunnel: [TRUE w581] -> w564
          tunnel: w563 -> [_ w580]
          tunnel: w555 -> [_ w579]
          frame False {
            w577 = FALSE  # rec
            # "counting AOD fill time"
          }
          frame True {
            w582 = TRUE  # rec
            w584 = u16 0  # Wait count
            # "AOD fill time reached"
            n122 = case shown="True" w579 {
              tunnel: [Image_State."Reference Scan" ("Enum") w587] -> w583
              tunnel: [TRUE ("Acquire MC") w588] -> w581
              tunnel: w580 -> [_ w589]
              frame False {
              }
              frame True {
                n123 = case shown="\"Pointing & MC\"" w589 {
                  tunnel: [Image_State."DAQ Scan" ("Enum") Image_State."DAQ Pointing" ("Enum") Image_State."DAQ Pointing" ("Enum") Image_State."DAQ Scan" ("Enum")] -> w587
                  tunnel: [FALSE FALSE FALSE FALSE] -> w588
                  frame "Scanning", Default {
                  }
                  frame "Pointing" {
                  }
                  frame "Pointing & MC" {
                  }
                  frame "Scanning & MC" {
                  }
                }
              }
            }
          }
        }
      }
    }
    n124 = case shown="True" w173 {
      tunnel: w98 -> [_ w602]
      tunnel: w97 -> [_ w601]
      tunnel: "select_ref_red" -> [_ w600]
      tunnel: w96 -> [_ w598]
      frame False {
      }
      frame True {
        # "ch1"
        # "ch0"
        # "write pixel ^ Acquire MC"
        n125 = Select(t=w602, s=w600, f=w601) -> (s? t:f=w599:u32)
        n126 = case "write ref pix (red = ch 0 green = ch1)" shown="True" w598 {
          tunnel: w599 -> [_ w603]
          frame False {
            # "Frame is incomplete"
          }
          frame True {
            # "Ref frame completed"
            n127 = xnode ("FIFO Method Node")("Element"=w603, "Timeout"=0) -> ()  [unwired: 1 in, 2 out]
          }
        }
      }
    }
    n128 = Add(x=w93, y=w92) -> (x+y=w85:dbl)
    n129 = Add(x=w91, y=w90) -> (x+y=w67:dbl)
    n130 = Add(x=w89, y=w88) -> (x+y=w65:dbl)
    n131 = Add(x=w87, y=w86) -> (x+y=w64:dbl)
    n132 = feedback #8() -> (w61:dbl)  [unwired: 1 in]
    n133 = feedback-in #8(w85) -> ()
    n134 = feedback #9() -> (w60:dbl)  [unwired: 1 in]
    n135 = feedback-in #9(w67) -> ()
    n136 = feedback #10() -> (w62:dbl)  [unwired: 1 in]
    n137 = feedback-in #10(w65) -> ()
    n138 = feedback #11() -> (w63:dbl)  [unwired: 1 in]
    n139 = feedback-in #11(w64) -> ()
    n140 = feedback #12() -> (w66:dbl)  [unwired: 1 in]
    n141 = feedback-in #12(w61) -> ()
    n142 = feedback #13() -> (w84:dbl)  [unwired: 1 in]
    n143 = feedback-in #13(w62) -> ()
    n144 = Subtract(x=w61, y=w60) -> (x-y=w72:dbl)
    n145 = Subtract(x=w60, y=w66) -> (x-y=w74:dbl)
    n146 = Subtract(x=w62, y=w63) -> (x-y=w79:dbl)
    n147 = Subtract(x=w63, y=w84) -> (x-y=w77:dbl)
    n148 = To Long Integer(number=w72) -> (32bit integer=w73:i32)
    n149 = To Long Integer(number=w74) -> (32bit integer=w75:i32)
    n150 = To Long Integer(number=w79) -> (32bit integer=w78:i32)
    n151 = To Long Integer(number=w77) -> (32bit integer=w76:i32)
    n152 = feedback #14() -> (w68:i32)  [unwired: 1 in]
    n153 = feedback-in #14(w73) -> ()
    n154 = feedback #15() -> (w69:i32)  [unwired: 1 in]
    n155 = feedback-in #15(w75) -> ()
    n156 = feedback #16() -> (w83:i32)  [unwired: 1 in]
    n157 = feedback-in #16(w78) -> ()
    n158 = feedback #17() -> (w82:i32)  [unwired: 1 in]
    n159 = feedback-in #17(w76) -> ()
    n160 = Absolute Value(x=w68) -> (abs(x)=w70:i32)
    n161 = Absolute Value(x=w69) -> (abs(x)=w71:i32)
    n162 = Absolute Value(x=w83) -> (abs(x)=w81:i32)
    n163 = Absolute Value(x=w82) -> (abs(x)=w80:i32)
    n164 = To Unsigned Long Integer(number=w70) -> (unsigned 32bit integer=w59:u32)
    n165 = To Unsigned Long Integer(number=w71) -> (unsigned 32bit integer=w58:u32)
    n166 = To Unsigned Long Integer(number=w81) -> (unsigned 32bit integer=w57:u32)
    n167 = To Unsigned Long Integer(number=w80) -> (unsigned 32bit integer=w56:u32)
    n168 = Add(x=w59, y=w58) -> (x+y=w101:u32)
    n169 = Add(x=w57, y=w56) -> (x+y=w100:u32)
  }
  n170 = timed-loop "Handshake loop" {
    timing: w29 -> [_]
    timing-out: [_] -> w28
    stop <- FALSE stop-if-true
    w641 = u8 32  # Data Length
    # "Used by the MC code in the PC code (\"Save MC Test Data.vi\"). Its value is saved to file.\nEliminate if unnecessary."
    # "Used by the MC code in the PC code (\"Save MC Test Data.vi\"). Its value is saved to file.\nEliminate if unnecessary."
    # "What does this really do?"
    # "Provide summary description of this loops functionality. What is it responsible for? Provide as many details as possible about the various individual signals and supply links/references to technical information where applicable. This can be anything (e.g. a website address, a document file's name, etc...)"
    # "What does this loop do??? Provide detailed description and enter loop title text above."
    # "HANDSHAKE LOOP"
    n171 = xnode ("FIFO Method Node")() -> ("Number of Elements to Read"=w625:u32, "FIFO Out"=w624:refnum<k21>)  [unwired: 1 in]
    n172 = Greater Than 0?(x=w625) -> (x > 0?=w623:bool)
    n173 = case shown="True" w623 {
      tunnel: w624 -> [_ w656]
      tunnel: [u32 0 ("Element") w659] -> w621
      tunnel: [FALSE TRUE] -> w618
      frame False {
      }
      frame True {
        n174 = xnode ("FIFO Method Node")("Timeout"=0, "FIFO In"=w656) -> ("Element"=w659:u32)  [unwired: 2 out]
      }
    }
    n175 = feedback #18(u32 0 ("Element")) -> (w622:u32)
    n176 = Select(t=w621, s=w618, f=w622) -> (s? t:f=w619:u32)
    "Read Value" <- w619
    n177 = feedback-in #18(w619) -> ()
    n178 = feedback #19() -> (w627:bool)  [unwired: 1 in]
    n179 = feedback-in #19(w618) -> ()
    n180 = Compound Arithmetic op=AND(w618, invert w627) -> (w635:bool)
    n181 = feedback #20 ("State")(SPI_Master_State."RESET") -> (w650:T12)
    n182 = feedback #21 ("CCount")() -> (w645:u8)  [unwired: 1 in]
    n183 = feedback #22 ("DCount")() -> (w644:u8)  [unwired: 1 in]
    n184 = feedback #23 ("SCLK")() -> (w643:bool)  [unwired: 1 in]
    n185 = feedback #24 ("Data Out")(u32 0 ("Data In")) -> (w626:u32)
    n186 = feedback #25 ("MOSI")() -> (w642:bool)  [unwired: 1 in]
    n187 = case shown="\"Assert MOSI\"" w650 {
      selector: w650 -> [_ w677 w689 w714 w730 w764]
      tunnel: [SPI_Master_State."Wait for TX" w670 w690 w715 w731 w765] -> w649
      tunnel: w635 -> [_ w666 _ _ _ _]
      tunnel: [w664 u8 0 w683 w708 w724 w759] -> w646
      tunnel: [w664 w672 w681 w707 w722 w747] -> w634
      tunnel: w645 -> [_ _ w686 w711 w727 w762]
      tunnel: w644 -> [_ _ w682 w707 w723 w747]
      tunnel: [TRUE ("MOSI") TRUE ("MOSI") _ _ _ _] -> w628
      tunnel: "CPHA" -> [_ w678 _ _ _ w753]
      tunnel: [w662 w671 w692 w703 w720 w755] -> w630
      tunnel: "CPOL" -> [w662 w671 _ _ _ _]
      tunnel: w643 -> [_ _ w692 w704 w721 w756]
      tunnel: w621 -> [_ w669 _ _ _ _]
      tunnel: [u32 0 ("Data In") w667 w695 w706 w735 w746] -> w632
      tunnel: w626 -> [_ w668 w696 w706 w736 w768]
      tunnel: "HCP-1" -> [_ _ w691 w716 w732 w766]
      tunnel: "MISO" -> [_ _ _ _ _ w757]
      tunnel: w641 -> [_ w672 _ _ _ _]
      tunnel: [FALSE ("msb carry out") w673 w694 w705 w734 w758] -> w616
      tunnel: w642 -> [_ w673 w693 w705 w733 w758]
      frame "RESET", Default {
        (unwired) FALSE ("msb carry out")
        w664 = u8 0
      }
      frame "Wait for TX" {
        n188 = Select(t=SPI_Master_State."Assert MOSI and Toggle SCLK", s=w678, f=SPI_Master_State."Assert MOSI" ("t")) -> (s? t:f=w674:T12)
        n189 = Select(t=w674, s=w666, f=w677) -> (s? t:f=w670:T12)
        n190 = Select(t=w669, s=w666, f=w668) -> (s? t:f=w667:u32)
      }
      frame "Assert MOSI" {
        n191 = Equal?(x=w691, y=w686) -> (x = y?=w687:bool)
        n192 = case shown="0" w686 {
          tunnel: w696 -> [w699 w701]
          tunnel: [w698 w701] -> w695
          tunnel: [w697 w702] -> w694
          tunnel: w693 -> [_ w702]
          frame 0 {
            n193 = Rotate Left With Carry(2:w699, 3:FALSE ("carry")) -> (0:w698:u32, 1:w697:bool)
          }
          frame 1, Default {
          }
        }
        n194 = Increment(x=w686) -> (x+1=w685:u8)
        n195 = Decrement(x=w682) -> (x-1=w681:u8)
        n196 = Select(t=u8 0, s=w687, f=w685) -> (s? t:f=w683:u8)
        n197 = Select(t=SPI_Master_State."Latch MISO and Toggle SCLK", s=w687, f=w689) -> (s? t:f=w690:T12)
      }
      frame "Toggle SCLK" {
        n198 = Equal?(x=w716, y=w711) -> (x = y?=w712:bool)
        n199 = case shown="1, Default" w711 {
          tunnel: w704 -> [w718 w719]
          tunnel: [w717 w719] -> w703
          frame 0 {
            n200 = Not(x=w718) -> (.not. x?=w717:bool)
          }
          frame 1, Default {
          }
        }
        n201 = Increment(x=w711) -> (x+1=w710:u8)
        n202 = Select(t=u8 0, s=w712, f=w710) -> (s? t:f=w708:u8)
        n203 = Select(t=SPI_Master_State."Wait for TX", s=w712, f=w714) -> (s? t:f=w715:T12)
      }
      frame "Assert MOSI and Toggle SCLK" {
        n204 = Equal?(x=w732, y=w727) -> (x = y?=w728:bool)
        n205 = case shown="0" w727 {
          tunnel: w736 -> [w737 w744]
          tunnel: [w741 w744] -> w735
          tunnel: [w740 w745] -> w734
          tunnel: w733 -> [_ w745]
          tunnel: w721 -> [w739 w743]
          tunnel: [w738 w743] -> w720
          frame 0 {
            n206 = Not(x=w739) -> (.not. x?=w738:bool)
            n207 = Rotate Left With Carry(2:w737, 3:FALSE ("carry")) -> (0:w741:u32, 1:w740:bool)
          }
          frame 1, Default {
          }
        }
        n208 = Increment(x=w727) -> (x+1=w726:u8)
        n209 = Decrement(x=w723) -> (x-1=w722:u8)
        n210 = Select(t=u8 0, s=w728, f=w726) -> (s? t:f=w724:u8)
        n211 = Select(t=SPI_Master_State."Latch MISO and Toggle SCLK", s=w728, f=w730) -> (s? t:f=w731:T12)
      }
      frame "Latch MISO and Toggle SCLK" {
        n212 = Equal?(x=w766, y=w762) -> (x = y?=w763:bool)
        n213 = Increment(x=w762) -> (x+1=w761:u8)
        n214 = case shown="0" w762 {
          tunnel: w768 -> [w776 w778]
          tunnel: [w772 w778] -> w767
          tunnel: w757 -> [w774 _]
          tunnel: w756 -> [w771 w777]
          tunnel: [w770 w777] -> w755
          frame 0 {
            n215 = Number To Boolean Array(number=w776) -> (Boolean array=w775:bool[])
            n216 = Not(x=w771) -> (.not. x?=w770:bool)
            n217 = Replace Array Subset(array=w775, new element=w774, index=0) -> (w773:bool[])
            n218 = Boolean Array To Number(Boolean array=w773) -> (number=w772:u32)
          }
          frame 1, Default {
          }
        }
        n219 = Equal To 0?(x=w747) -> (x = 0?=w754:bool)
        n220 = Select(t=u8 0, s=w763, f=w761) -> (s? t:f=w759:u8)
        n221 = Select(t=SPI_Master_State."Wait for TX", s=w753, f=SPI_Master_State."Toggle SCLK" ("t")) -> (s? t:f=w749:T12)
        n222 = Select(t=w749, s=w754, f=SPI_Master_State."Assert MOSI and Toggle SCLK" ("t")) -> (s? t:f=w751:T12)
        n223 = Select(t=w751, s=w763, f=w764) -> (s? t:f=w765:T12)
        n224 = To Unsigned Long Integer(number=w767) -> (unsigned 32bit integer=w746:u32)
      }
    }
    "_SS" <- w628
    "Data Out" <- w632
    n225 = feedback-in #21(w646) -> ()
    n226 = feedback-in #22(w634) -> ()
    n227 = feedback-in #23(w630) -> ()
    n228 = feedback-in #24(w632) -> ()
    n229 = feedback-in #25(w616) -> ()
    n230 = Build Array(w628, w630, w616) -> (w631:bool[])
    n231 = Boolean Array To Number(Boolean array=w631) -> (number=w653:u8)
    n232 = xnode "FPGA I/O Node"("IO Module\\DIO Port 0 Wr Data"=w653, "IO Module\\DIO Port 0 WE Request"=TRUE ("IO Module\\DIO Port 0 WE Request"), "IO Module\\DIO Port 1 WE Request"=FALSE ("IO Module\\DIO Port 1 WE Request")) -> ()  [unwired: 3 in, 3 out]
    n233 = Select(t=SPI_Master_State."RESET", s="RESET", f=w649) -> (s? t:f=w636:T12)
    n234 = feedback-in #20(w636) -> ()
  }
  n235 = timed-loop "Timed Loop" {
    timing: w5 -> [_]
    timing-out: [_] -> w4
    stop <- FALSE stop-if-true
    # "Used by the MC code in the PC code (\"Save MC Test Data.vi\"). Its value is saved to file.\nEliminate if unnecessary."
    # "Used by the MC code in the PC code (\"Save MC Test Data.vi\"). Its value is saved to file.\nEliminate if unnecessary."
    # "Used by the MC code in the PC code (\"Save MC Test Data.vi\"). Its value is saved to file.\nEliminate if unnecessary."
    # "first frame"
    # "capture ref"
    # "Missing pipelining\nshift register?"
    # "Detects a rising edge on the \"Trigger In\" signal"
    # "Zero if > threshold"
    # "last pixel"
    # "last pixel"
    # "increment y"
    # "increment x"
    # "Missing pipelining\nshift register?"
    # "Initialise?"
    # "Initialise?"
    # "Input valid"
    # "Last pixel"
    # "This looks redundant"
    # "This looks redundant"
    # "This looks redundant"
    # "Provide a summary of this loop's purpose and functionality, and enter loop title text above."
    # "Eliminate indicators when no longer needed"
    # "Eliminate indicators when no longer needed"
    # "NB swaped subtraction to negate x for Geoff's code scanning in opposite x"
    # "scale by * 1-2"
    # "I32*dwelltime(us)/100 = (I32*refsnmps*5)/1000*100 = I32*refsmaple/20000"
    # "set from host"
    # "sum_ys"
    # "sum_xs"
    # "sumall"
    # "<Title Goes Here>"
    n236 = global read "FPGA golbals.vi" "Trigger In"() -> (w784:bool)
    n237 = xnode ("FIFO Method Node")() -> ("Number of Elements to Read"=w1030:u32, "FIFO Out"=w1029:refnum<k21>)  [unwired: 1 in]
    n238 = global read "FPGA golbals.vi" "MC"() -> (w783:bool)
    n239 = And(x=w784, y=w783) -> (x .and. y?=w794:bool)
    n240 = feedback #26(FALSE) -> (w795:bool)
    n241 = feedback-in #26(w794) -> ()
    n242 = local read "Ref samps-per-pix (Pr)"() -> (w894:u16)
    n243 = Compound Arithmetic op=AND(w794, invert w795) -> (w793:bool)
    n244 = Greater Than 0?(x=w1030) -> (x > 0?=w1027:bool)
    n245 = feedback #27(FALSE) -> (w868:bool)
    n246 = And(x=w1027, y=w868) -> (x .and. y?=w866:bool)
    n247 = case shown="True" w866 {
      tunnel: w1029 -> [_ w1165]
      tunnel: [0 ("Element") w1164] -> w1028
      tunnel: [FALSE TRUE] -> w941
      frame False {
      }
      frame True {
        n248 = xnode ("FIFO Method Node")("Timeout"=0, "FIFO In"=w1165) -> ("Element"=w1164:i32)  [unwired: 2 out]
      }
    }
    n249 = feedback #28 ("MC State")(first_ref_frame."Waiting") -> (w948:T2)
    n250 = To Fixed-Point(number=w894) -> (fixed-point=w942:fxp<+,16,16>)  [unwired: 1 in]
    n251 = xnode ("High Throughput Multiply")("x"=w942, "y"=fxp<+,16,16> 2.0) -> ("x*y"=w938:fxp<+,16,16>)
    n252 = To Unsigned Long Integer(number=w1028) -> (unsigned 32bit integer=w944:u32)
    n253 = To Fixed-Point(number=w944) -> (fixed-point=w939:fxp<+,32,32>)  [unwired: 1 in]
    n254 = local read "Ref x-pixels-per-line (Npxr)"() -> (w893:i16)
    n255 = local read "Ref y-pixels-per-line (Npyr)"() -> (w892:i16)
    n256 = feedback #29(u16 1 ("t")) -> (w1010:u16)
    n257 = Increment(x=w1010) -> (x+1=w1012:u16)
    n258 = feedback #30(u16 0 ("t")) -> (w994:u16)
    n259 = Increment(x=w994) -> (x+1=w1022:u16)
    n260 = feedback #31(u16 0 ("t")) -> (w961:u16)
    n261 = feedback #32(u16 1 ("t")) -> (w802:u16)
    n262 = feedback #33(u16 0 ("t")) -> (w947:u16)
    n263 = feedback #34(FALSE ("dv in")) -> (w799:bool)
    n264 = To Unsigned Word Integer(number=w892) -> (unsigned 16bit integer=w928:u16)
    n265 = To Unsigned Word Integer(number=w893) -> (unsigned 16bit integer=w929:u16)
    n266 = case shown="True" w799 {
      tunnel: w947 -> [_ w1073]
      frame False {
      }
      frame True {
        # "Debug FIFO for reference data"
        n267 = xnode ("FIFO Method Node")("Element"=w1073, "Timeout"=0) -> ()  [unwired: 1 in, 2 out]
      }
    }
    n268 = To Fixed-Point(number=w947) -> (fixed-point=w1015:fxp<+,16,16>)  [unwired: 1 in]
    n269 = Equal?(x=w929, y=w961) -> (x = y?=w796:bool)
    n270 = Equal?(x=w802, y=w928) -> (x = y?=w964:bool)
    n271 = Select(t=w1015, s=w799, f=fxp<+,16,16> 0.0) -> (s? t:f=w1018:fxp<+,16,16>)
    n272 = case shown="True" w799 {
      tunnel: w961 -> [_ w1153]
      tunnel: w1015 -> [_ w1155]
      tunnel: [fxp<+,32,32> 0.0 ("x*y") w1158] -> w1014
      tunnel: w802 -> [_ w1156]
      tunnel: [fxp<+,32,32> 0.0 ("x*y") w1154] -> w1013
      frame False {
      }
      frame True {
        n273 = To Fixed-Point(number=w1153) -> (fixed-point=w1159:fxp<+,16,16>)  [unwired: 1 in]
        n274 = To Fixed-Point(number=w1156) -> (fixed-point=w1157:fxp<+,16,16>)  [unwired: 1 in]
        n275 = xnode ("High Throughput Multiply")("x"=w1155, "y"=w1157) -> ("x*y"=w1154:fxp<+,32,32>)
        n276 = xnode ("High Throughput Multiply")("x"=w1155, "y"=w1159) -> ("x*y"=w1158:fxp<+,32,32>)
      }
    }
    n277 = feedback #35(fxp<+,32,32> data[16B] ("x+y")) -> (w845:fxp<+,32,32>)
    n278 = feedback #36(FALSE ("dv in")) -> (w989:bool)
    n279 = feedback-in #36(w799) -> ()
    n280 = feedback #37(fxp<+,32,32> data[16B] ("x+y")) -> (w1009:fxp<+,32,32>)
    n281 = feedback #38(fxp<+,32,32> 0.0 ("x*y")) -> (w1006:fxp<+,32,32>)
    n282 = feedback-in #38(w1014) -> ()
    n283 = feedback #39(fxp<+,32,32> 0.0 ("x*y")) -> (w1001:fxp<+,32,32>)
    n284 = feedback-in #39(w1013) -> ()
    n285 = Select(t=w1006, s=w989, f=fxp<+,16,16> 0.0) -> (s? t:f=w1007:fxp<+,32,32>)
    n286 = Select(t=w1001, s=w989, f=fxp<+,16,16> 0.0) -> (s? t:f=w1003:fxp<+,32,32>)
    n287 = feedback #40(FALSE ("dv in")) -> (w800:bool)
    n288 = feedback-in #40(w989) -> ()
    n289 = feedback #41(fxp<+,32,32> data[16B] ("x+y")) -> (w951:fxp<+,32,32>)
    n290 = feedback #42(fxp<+,32,32> data[16B] ("x+y")) -> (w956:fxp<+,32,32>)
    n291 = Compound Arithmetic op=AND(w800, w796) -> (w803:bool)
    n292 = Select(t=u16 0, s=w803, f=w994) -> (s? t:f=w995:u16)
    n293 = Select(t=w1012, s=w803, f=w1010) -> (s? t:f=w992:u16)
    n294 = Compound Arithmetic op=AND(w800, w796, w964) -> (w798:bool)
    n295 = Select(t=u16 1, s=w798, f=w992) -> (s? t:f=w991:u16)
    n296 = feedback-in #29(w991) -> ()
    n297 = feedback-in #32(w991) -> ()
    n298 = Select(t=fxp<+,32,32> data[16B], s=w798, f=w845) -> (s? t:f=w949:fxp<+,32,32>)
    n299 = xnode ("High Throughput Add")("x"=w1018, "y"=w949) -> ("x+y"=w1019:fxp<+,32,32>)  [unwired: 1 out]
    n300 = feedback-in #35(w1019) -> ()
    n301 = feedback-in #37(w1019) -> ()
    n302 = Select(t=fxp<+,32,32> data[16B], s=w798, f=w951) -> (s? t:f=w952:fxp<+,32,32>)
    n303 = Select(t=fxp<+,32,32> data[16B], s=w798, f=w956) -> (s? t:f=w957:fxp<+,32,32>)
    n304 = xnode ("High Throughput Add")("x"=w1007, "y"=w952) -> ("x+y"=w958:fxp<+,32,32>)  [unwired: 1 out]
    n305 = xnode ("High Throughput Add")("x"=w1003, "y"=w957) -> ("x+y"=w1004:fxp<+,32,32>)  [unwired: 1 out]
    n306 = feedback-in #41(w958) -> ()
    n307 = feedback-in #42(w1004) -> ()
    n308 = feedback #43(fxp<+,32,32> data[16B] ("x+y")) -> (w999:fxp<+,32,32>)
    n309 = feedback-in #43(w1004) -> ()
    n310 = feedback #44(fxp<+,32,32> data[16B] ("x+y")) -> (w998:fxp<+,32,32>)
    n311 = feedback-in #44(w1009) -> ()
    n312 = feedback #45(fxp<+,32,32> data[16B] ("x+y")) -> (w1000:fxp<+,32,32>)
    n313 = feedback-in #45(w958) -> ()
    n314 = xnode "High Throughput Divide"("x"=w1000, "y"=w998, "input valid"=w798) -> ("x/y"=w891:fxp<+,32,16>, "output valid"=w886:bool, "ready for input"=w997:bool)  [unwired: 1 in]
    n315 = xnode "High Throughput Divide"("x"=w999, "y"=w998, "input valid"=w798) -> ("x/y"=w889:fxp<+,32,16>, "output valid"=w887:bool, "ready for input"=w996:bool)  [unwired: 1 in]
    n316 = call "average_centroid.vi"("input valid"=w886, "Average"="Average", "Input value"=w891) -> ("av_ready"=w805:bool, "cent_av"=w890:fxp<+,32,16>)  [unwired: 7 in]
    n317 = call "average_centroid.vi"("input valid"=w887, "Average"="Average", "Input value"=w889) -> ("av_ready"=w809:bool, "cent_av"=w888:fxp<+,32,16>)  [unwired: 7 in]
    n318 = And(x=w997, y=w996) -> (x .and. y?=w869:bool)
    n319 = xnode "High Throughput Divide"("x"=w939, "y"=w938, "input valid"=w941, "ready for output (T)"=w869) -> ("x/y"=w940:fxp<+,16,16>, "output valid"=w797:bool, "ready for input"=w867:bool)
    n320 = feedback-in #27(w867) -> ()
    n321 = To Unsigned Word Integer(number=w940) -> (unsigned 16bit integer=w846:u16)
    n322 = Less?(x=w846, y="threshold") -> (x < y?=w1025:bool)
    n323 = Select(t=w1022, s=w797, f=w995) -> (s? t:f=w1020:u16)
    n324 = feedback-in #30(w1020) -> ()
    n325 = Select(t=u16 0, s=w1025, f=w846) -> (s? t:f=w1024:u16)
    n326 = feedback-in #31(w1020) -> ()
    n327 = feedback-in #33(w1024) -> ()
    n328 = feedback-in #34(w797) -> ()
    n329 = feedback #46(FALSE) -> (w815:bool)
    n330 = case shown="\"Wrote Ref\"" w948 {
      tunnel: w793 -> [w1080 _ _]
      tunnel: [w1079 w1085 w1089] -> w988
      tunnel: w815 -> [_ w1086 _]
      tunnel: [w1077 w1084 w1087] -> w925
      tunnel: [w1078 w1083 w1092] -> w924
      tunnel: w783 -> [_ _ w1091]
      frame "Waiting", Default {
        w1077 = FALSE  # first frame
        w1078 = TRUE  # No ref
        n331 = Select(t=first_ref_frame."First frame", s=w1080, f=first_ref_frame."Waiting") -> (s? t:f=w1079:T2)
      }
      frame "First frame" {
        w1083 = TRUE  # No ref
        w1084 = TRUE  # first frame
        n332 = Select(t=first_ref_frame."Wrote Ref", s=w1086, f=first_ref_frame."First frame") -> (s? t:f=w1085:T2)
      }
      frame "Wrote Ref" {
        w1087 = TRUE  # first frame
        w1092 = FALSE  # No ref
        n333 = Select(t=first_ref_frame."Wrote Ref", s=w1091, f=first_ref_frame."Waiting") -> (s? t:f=w1089:T2)
      }
    }
    "MC State" <- w988
    n334 = feedback-in #28(w988) -> ()
    n335 = And(x="set_reference", y=w925) -> (x .and. y?=w885:bool)
    n336 = And(x=w885, y=w805) -> (x .and. y?=w923:bool)
    n337 = And(x=w809, y=w885) -> (x .and. y?=w808:bool)
    n338 = feedback-in #46(w808) -> ()
    n339 = feedback #47 ("x_centroid_ref")(fxp<+,32,16> data[16B] ("x/y")) -> (w855:fxp<+,32,16>)
    "x_centroid_ref" <- w855
    n340 = Select(t=w890, s=w923, f=w855) -> (s? t:f=w986:fxp<+,32,16>)
    n341 = feedback-in #47(w986) -> ()
    n342 = feedback #48(fxp<+,32,16> data[16B] ("x/y")) -> (w853:fxp<+,32,16>)
    n343 = Select(t=w890, s=w805, f=w853) -> (s? t:f=w982:fxp<+,32,16>)
    n344 = feedback-in #48(w982) -> ()
    n345 = feedback #49(FALSE ("dv in")) -> (w804:bool)
    "x_new_ready" <- w804
    n346 = feedback-in #49(w805) -> ()
    n347 = feedback #50 "y_centroid_new"(fxp<+,32,16> data[16B] ("x/y")) -> (w962:fxp<+,32,16>)
    "y_centroid_new" <- w962
    n348 = Select(t=w888, s=w809, f=w962) -> (s? t:f=w980:fxp<+,32,16>)
    n349 = feedback-in #50(w980) -> ()
    n350 = feedback #51 "y_centroid_ref"(fxp<+,32,16> data[16B] ("x/y")) -> (w963:fxp<+,32,16>)
    "y_centroid_ref" <- w963
    n351 = Select(t=w888, s=w808, f=w963) -> (s? t:f=w985:fxp<+,32,16>)
    n352 = feedback-in #51(w985) -> ()
    n353 = feedback #52(FALSE ("dv in")) -> (w932:bool)
    "y_new_ready" <- w932
    n354 = feedback-in #52(w809) -> ()
    n355 = feedback #53() -> (w852:fxp<+,32,16>)  [unwired: 1 in]
    n356 = Select(t=w853, s=w804, f=w852) -> (s? t:f=w851:fxp<+,32,16>)
    "x_centroid_new" <- w851
    n357 = feedback-in #53(w851) -> ()
    n358 = To Fixed-Point(number=w855) -> (fixed-point=w880:fxp<+,32,16>)  [unwired: 1 in]
    n359 = To Fixed-Point(number=w853) -> (fixed-point=w881:fxp<+,32,16>)  [unwired: 1 in]
    n360 = To Fixed-Point(number=w962) -> (fixed-point=w978:fxp<+,32,16>)  [unwired: 1 in]
    n361 = To Fixed-Point(number=w963) -> (fixed-point=w977:fxp<+,32,16>)  [unwired: 1 in]
    n362 = xnode ("High Throughput Subtract")("x"=w978, "y"=w977, "input valid"=w932) -> ("x-y"=w919:fxp<+/-,16,8>, "output valid"=w931:bool)  [unwired: 1 in, 1 out]
    n363 = xnode ("High Throughput Subtract")("x"=w880, "y"=w881, "input valid"=w804) -> ("x-y"=w883:fxp<+/-,16,8>, "output valid"=w933:bool)  [unwired: 1 in, 1 out]
    n364 = Or(x=w923, y=w924) -> (x .or. y?=w850:bool)
    n365 = Or(x=w808, y=w924) -> (x .or. y?=w816:bool)
    n366 = feedback #54(fxp<+/-,16,8> data[16B] ("x-y")) -> (w801:fxp<+/-,16,8>)
    n367 = feedback-in #54(w883) -> ()
    n368 = feedback #55(FALSE ("dv in")) -> (w879:bool)
    n369 = feedback-in #55(w933) -> ()
    n370 = feedback #56(fxp<+/-,16,8> data[16B] ("x-y")) -> (w834:fxp<+/-,16,8>)
    n371 = feedback-in #56(w919) -> ()
    n372 = feedback #57(FALSE ("dv in")) -> (w878:bool)
    n373 = feedback-in #57(w931) -> ()
    n374 = Absolute Value(x=w801) -> (abs(x)=w836:fxp<+,16,8>)
    n375 = Absolute Value(x=w834) -> (abs(x)=w841:fxp<+,16,8>)
    n376 = Greater?(x=w841, y=fxp<+/-,16,8> data[16B] ("x")) -> (0:w844:bool)
    n377 = Greater?(x=w836, y=fxp<+/-,16,8> data[16B] ("x")) -> (0:w839:bool)
    n378 = Select(t=fxp<+/-,16,8> data[17B], s=w839, f=w801) -> (s? t:f=w835:fxp<+/-,16,8>)
    "x_diff" <- w835
    n379 = Select(t=fxp<+/-,16,8> data[17B], s=w844, f=w834) -> (s? t:f=w840:fxp<+/-,16,8>)
    "y_diff" <- w840
    n380 = feedback-in #58(w878) -> ()
    n381 = feedback #58(FALSE ("dv in")) -> (w811:bool)
    n382 = feedback-in #59(w879) -> ()
    n383 = feedback #59(FALSE ("dv in")) -> (w812:bool)
    n384 = call "thresh_diff.vi"("diff_thresh"="diff_thresh", "x_diff in"=w835) -> ("thresh_out"=w874:fxp<+/-,16,8>)  [unwired: 9 in]
    n385 = call "thresh_diff.vi"("diff_thresh"="diff_thresh", "x_diff in"=w840) -> ("thresh_out"=w873:fxp<+/-,16,8>)  [unwired: 9 in]
    n386 = To Fixed-Point(fixed-point type=fxp<+,16,1> 0.0, number="scan_int") -> (fixed-point=w820:fxp<+,16,1>)
    n387 = call "PI_controller_dt.vi"("dv in"=w812, "xy_diff_in"=w874, "scan_int"="scan_int", "write_first_centroid"=w850, "proportional"="proportioanl_scale", "Intmult"="Integral_scale") -> ("xydiffvalid"=w861:bool, "xydiff_out"=w860:fxp<+/-,16,8>)  [unwired: 4 in]
    "xpiddiffvalid" <- w861
    n388 = call "PI_controller_dt.vi"("dv in"=w811, "xy_diff_in"=w873, "scan_int"="scan_int", "write_first_centroid"=w816, "proportional"="proportioanl_scale", "Intmult"="Integral_scale") -> ("xydiffvalid"=w813:bool, "xydiff_out"=w877:fxp<+/-,16,8>)  [unwired: 4 in]
    "y_diff_PID_out" <- w877
    "ydiffpidvalid" <- w813
    n389 = feedback #60() -> (w859:fxp<+/-,16,8>)  [unwired: 1 in]
    n390 = Select(t=w860, s=w861, f=w859) -> (s? t:f=w854:fxp<+/-,16,8>)
    "x_diff_PID_out" <- w854
    n391 = feedback-in #60(w854) -> ()
    n392 = feedback #61(fxp<+/-,16,8> data[16B] ("x+y")) -> (w910:fxp<+/-,16,8>)
    n393 = feedback #62(FALSE ("dv in")) -> (w971:bool)
    n394 = feedback #63(fxp<+/-,16,8> data[16B] ("x+y")) -> (w908:fxp<+/-,16,8>)
    n395 = feedback #64(FALSE ("dv in")) -> (w966:bool)
    n396 = feedback #65(fxp<+/-,16,8> data[16B] ("t")) -> (w973:fxp<+/-,16,8>)
    n397 = xnode ("High Throughput Add")("x"=w973, "y"=w860, "input valid"=w861) -> ("x+y"=w911:fxp<+/-,16,8>, "output valid"=w863:bool)  [unwired: 1 in, 1 out]
    n398 = feedback-in #61(w911) -> ()
    n399 = feedback-in #62(w863) -> ()
    n400 = Select(t=fxp<+/-,16,8> data[16B], s=w850, f=w973) -> (s? t:f=w974:fxp<+/-,16,8>)
    n401 = disable-structure shown="Disabled" {
      disable-tunnel: w863 -> [w1041 _]
      disable-tunnel: w799 -> [w1032 _]
      frame Disabled {
        # "Debugging code. Add an indicator to\nview the value."
        n402 = feedback #66(u32 0 ("t")) -> (w1040:u32)
        n403 = feedback #67(u32 0) -> (w1037:u32)
        n404 = Select(t=w1037, s=w1032, f=w1040) -> (s? t:f=w1035:u32)
        n405 = Select(t=u32 0, s=w1041, f=w1035) -> (s? t:f=w1033:u32)
        n406 = feedback-in #66(w1033) -> ()
        n407 = Increment(x=w1033) -> (x+1=w1039:u32)
        n408 = feedback-in #67(w1039) -> ()
      }
      frame Enabled {
      }
    }
    n409 = feedback #68(FALSE ("dv in")) -> (w830:bool)
    n410 = feedback-in #68(w971) -> ()
    n411 = feedback #69(fxp<+/-,16,8> data[16B] ("t")) -> (w968:fxp<+/-,16,8>)
    n412 = xnode ("High Throughput Add")("x"=w968, "y"=w877, "input valid"=w813) -> ("x+y"=w909:fxp<+/-,16,8>, "output valid"=w930:bool)  [unwired: 1 in, 1 out]
    n413 = feedback-in #63(w909) -> ()
    n414 = feedback-in #64(w930) -> ()
    n415 = Select(t=fxp<+/-,16,8> data[16B], s=w816, f=w968) -> (s? t:f=w969:fxp<+/-,16,8>)
    n416 = feedback #70(FALSE ("dv in")) -> (w828:bool)
    n417 = feedback-in #70(w966) -> ()
    n418 = Select(t=w910, s=w971, f=w974) -> (s? t:f=w858:fxp<+/-,16,8>)
    n419 = feedback-in #65(w858) -> ()
    n420 = Select(t=w908, s=w966, f=w969) -> (s? t:f=w907:fxp<+/-,16,8>)
    n421 = feedback-in #69(w907) -> ()
    n422 = Or(x=w830, y=w828) -> (x .or. y?=w831:bool)
    n423 = feedback #71 "x_offset"(fxp<+/-,16,8> data[16B] ("t")) -> (w819:fxp<+/-,16,8>)
    n424 = feedback-in #71(w858) -> ()
    n425 = feedback #72 "y_offset"(fxp<+/-,16,8> data[16B] ("t")) -> (w789:fxp<+/-,16,8>)
    n426 = feedback-in #72(w907) -> ()
    n427 = call "kalman_int_v3.vi"("y_offset"=w789, "x_offset"=w819, "reset"=w816, "new_offset"=w831, "var_x"="var_x", "var_y"="var_y", "accn_noise"="accn_noise", "feedback_time (ms)"=w820) -> ("q2_ready"=w829:bool, "Q2_update"=w791:fxp<+/-,16,8>, "q1_ready"=w833:bool, "Q1_update"=w832:fxp<+/-,16,8>)
    n428 = Select(t=w832, s="use Kalman", f=w819) -> (s? t:f=w818:fxp<+/-,16,8>)
    n429 = Select(t=w791, s="use Kalman", f=w789) -> (s? t:f=w790:fxp<+/-,16,8>)
    n430 = Select(t=w833, s="use Kalman", f=w830) -> (s? t:f=w817:bool)
    n431 = Select(t=w829, s="use Kalman", f=w828) -> (s? t:f=w827:bool)
    n432 = Select(t="x_offset_host", s="use host offset", f=w818) -> (s? t:f=w862:fxp<+/-,16,8>)
    n433 = Select(t="y_offset_host", s="use host offset", f=w790) -> (s? t:f=w884:fxp<+/-,16,8>)
    "y_offset" <- w884
    n434 = feedback #73 "x_offset"() -> (w782:fxp<+/-,16,8>)  [unwired: 1 in]
    n435 = Select(t=w862, s=w817, f=w782) -> (s? t:f=w781:fxp<+/-,16,8>)
    "x_offset" <- w781
    n436 = feedback-in #73(w781) -> ()
    n437 = xnode ("High Throughput Multiply")("x"="scale", "y"=w862, "input valid"=w817) -> ("x*y"=w897:fxp<+/-,16,8>, "output valid"=w872:bool)  [unwired: 1 in, 1 out]
    n438 = xnode ("High Throughput Multiply")("x"="scale", "y"=w884, "input valid"=w827) -> ("x*y"=w895:fxp<+/-,16,8>, "output valid"=w871:bool)  [unwired: 1 in, 1 out]
    n439 = And(x=w872, y=w871) -> (x .and. y?=w814:bool)
    n440 = Number To Boolean Array(number=w897) -> (Boolean array=w903:bool[])
    n441 = Number To Boolean Array(number=w895) -> (Boolean array=w900:bool[])
    n442 = And(x=w814, y=w783) -> (x .and. y?=w848:bool)
    "TX ready" <- w848
    n443 = Boolean Array To Number(Boolean array=w903) -> (number=w857:u16)
    "x_offset_u16" <- w857
    n444 = Boolean Array To Number(Boolean array=w900) -> (number=w898:u16)
    "y_offset_u16" <- w898
    n445 = Join Numbers(hi=w898, lo=w857) -> ((hi.lo)=w899:u32)
    n446 = feedback-in #74(w848) -> ()
    n447 = feedback #74(bool[] [FALSE, FALSE, FALSE]) -> (w849:bool)
    n448 = feedback #75(u32 0) -> (w865:u32)
    n449 = Select(t=w899, s=w814, f=w865) -> (s? t:f=w870:u32)
    "y^x offset" <- w870
    n450 = case shown="True" w849 {
      tunnel: w865 -> [_ w1043]
      frame False {
      }
      frame True {
        n451 = xnode ("FIFO Method Node")("Element"=w1043, "Timeout"=0) -> ()  [unwired: 1 in, 2 out]
      }
    }
    n452 = feedback-in #75(w870) -> ()
  }
  n453 = node-c288(w2) -> ()
  n454 = node-c288(w28) -> ()
  n455 = node-c288(w26) -> ()
  n456 = node-c288(w4) -> ()
